vi "运维调试_CODMn.vi"() -> ()   [LabVIEW 2016, in "斯坦道CODMn新电路板.lvlib"]
uses:
  <vilib>/Utility/miscctls.llb/LVPointTypeDef.ctl
  <vilib>/Waveform/WDTFileIO.llb/Read Waveform from File.vi
  <vilib>/Utility/config.llb/NI_LVConfig.lvlib
  <vilib>/ptbypt/NI_PtbyPt.lvlib
panel:
  in  "量程下拉列表 2":enum16{"低量程", "高量程"}(ring)
  out "消解压力kPa":sgl format="%#.2f"
  out "权限等级":string
  out "总步数":i32
  out "滑动杆":u8(slide) caption="测试进度" scale=0.0..100.0
  in  "参数查询":bool
  in  "仪器校准":bool
  out "仪器版本号":string
  in  "试剂余量设置":bool
  out "试剂余量显示":sgl[][](graph)
  in  "公式切换阈值滴定数(0~9999)":dbl
  out "X0":u16
  in  "平台反控标样校准":enum16{"标液1", "标液2", "标液3"}(ring)
  in  "平台反控校准量程":enum16{"低量程1", "低量程2", "高量程1", "高量程2"}(ring)
  out "注射泵保温温度":sgl format="%#.2f"
  out "量程参数显示":T1 {"(高->低)" format="%#.6g"; "阈值(低->高)" format="%#.6g"; "下限" format="%#.6g"; "上限" format="%#.6g"}
  in  "历史波形 2":bool
  in  "返回 3":bool
  out "时间-温度":u16[](array[numeric]) caption="数组"
  out "温度波形时间":timestamp
  out "ORP滴定曲线 2":u16[](graph)
  in  "历史波形":bool
  in  "返回 2":bool
  out "滴定数-ORP值":u16[](array[numeric]) caption="数组"
  out "波形时间":timestamp
  out "ORP滴定曲线":u16[](graph)
  in  "滴定曲线":bool
  out "终点滴定数":sgl format="%#.2f"
  out "单位:":T2(ring)
  out "运行状态":T3 {"数据时间:" format="%<%y/%m/%d %H:%M:%S>T"; "仪器时间:" format="%<%y/%m/%d %H:%M:%S>T"}
  out "模块版本号":string
  in  "模型选择":cluster{"参数":u8, "测量模式":u8, "量程":u8}
  in  "校准完毕":bool
  in  "校准按钮":T4
  in  "曲线模型":T5={"标液浓度1"=0.0, "测量吸光度1"=0.0, "样品1启用"=FALSE, "标液浓度2"=0.0, "测量吸光度2"=0.0, "样品2启用"=FALSE, "标液浓度3"=0.0, "测量吸光度3"=0.0, "样品3启用"=FALSE, "标液浓度4"=0.0, "测量吸光度4"=0.0, "样品4启用"=FALSE, "标液浓度5"=0.0, "测量吸光度5"=0.0, "样品5启用"=FALSE, "模型"=enum."线性", "method"=enum."最小二乘", "精度"=7.0, "XY图"=[], "拟合公式"="", "r^2"=0.0, "零点校准时间"=timestamp(0 s since 1904-01-01), "标液校准时间1"=timestamp(0 s since 1904-01-01), "标液校准时间2"=timestamp(0 s since 1904-01-01), "标液校准时间3"=timestamp(0 s since 1904-01-01), "标液校准时间4"=timestamp(0 s since 1904-01-01)} {"标液校准时间4" format="%<%Y/%m/%d %H:%M:%S>T"; "标液校准时间3" format="%<%Y/%m/%d %H:%M:%S>T"; "标液校准时间2" format="%<%Y/%m/%d %H:%M:%S>T"; "标液校准时间1" format="%<%Y/%m/%d %H:%M:%S>T"; "零点校准时间" format="%<%Y/%m/%d %H:%M:%S>T"; "r^2" format="%.7g"; "标液浓度5" format="%#.2f"; "测量吸光度5" format="%#.0f"; "标液浓度4" format="%#.2f"; "测量吸光度4" format="%#.0f"; "标液浓度3" format="%#.2f"; "测量吸光度3" format="%#.0f"; "标液浓度2" format="%#.2f"; "测量吸光度2" format="%#.0f"; "测量吸光度1" format="%#.0f"; "标液浓度1" format="%#.2f"}
  out "公式、校准输出":T6={"公式"={"X^2"=0.0, "X"=nan, "B"=nan}, "校准"={"校准？"=FALSE, "校准点1-5"=0, "校准浓度"=0.0}}
  out "当前步骤剩余时间":sgl format="%#.2f"
  out "加热实时温度":sgl format="%#.2f"
  out "ORP值/光值":sgl format="%#.2f"
  in  "布尔":bool
  in  "流程固件":bool
  in  "公式单个写入":bool
  in  "流程路径":path=path "C:/Users/STD/Documents/斯坦道流程文件/流程.xml"
  out "字符串":string
  out "运行时间":sgl format="%#.2f"
  out "环境湿度":sgl format="%#.2g"
  out "环境温度":sgl format="%#.2g"
  out "固件版本号":string
  in  "数组":string[](array[string])
  in  "量程切换阈值写入":bool
  in  "量程切换阈值读取":bool
  in  "参数下拉列表":enum16{"CODMn"}(ring)
  in  "量程下拉列表":enum16{"低量程1", "低量程2", "高量程1", "高量程2"}(ring)
  in  "测量模式下拉列表":T7(ring)=enum."水样测量"
  in  "公式":cluster{"X^2":dbl, "X":dbl, "b":dbl}
  in  "写公式":bool
  in  "读公式":bool
  in  "返回":bool
  in  "设置":bool
  out "集成报警信息":string
  in  "定时启动":cluster{"启动":bool, "控制命令":T8, "测量参数":T9}(xcontrol)
  in  "停止":bool
  in  "手动启动":bool
  in  "单步测试":bool
  out "当前滴定数":sgl format="%#.2f"
  out "K":sgl format="%#.2f"
  out "B":sgl format="%#.2f"
  out "A":sgl format="%#.2f"
  out "多列列表框":i32(listbox)
  # "."
  # "校准时间"
  # "标液浓度"
  # "滴定数显示"
  # "标液1"
  # "标液2"
  # "标液3"
  # "零点"
  # "跨度"
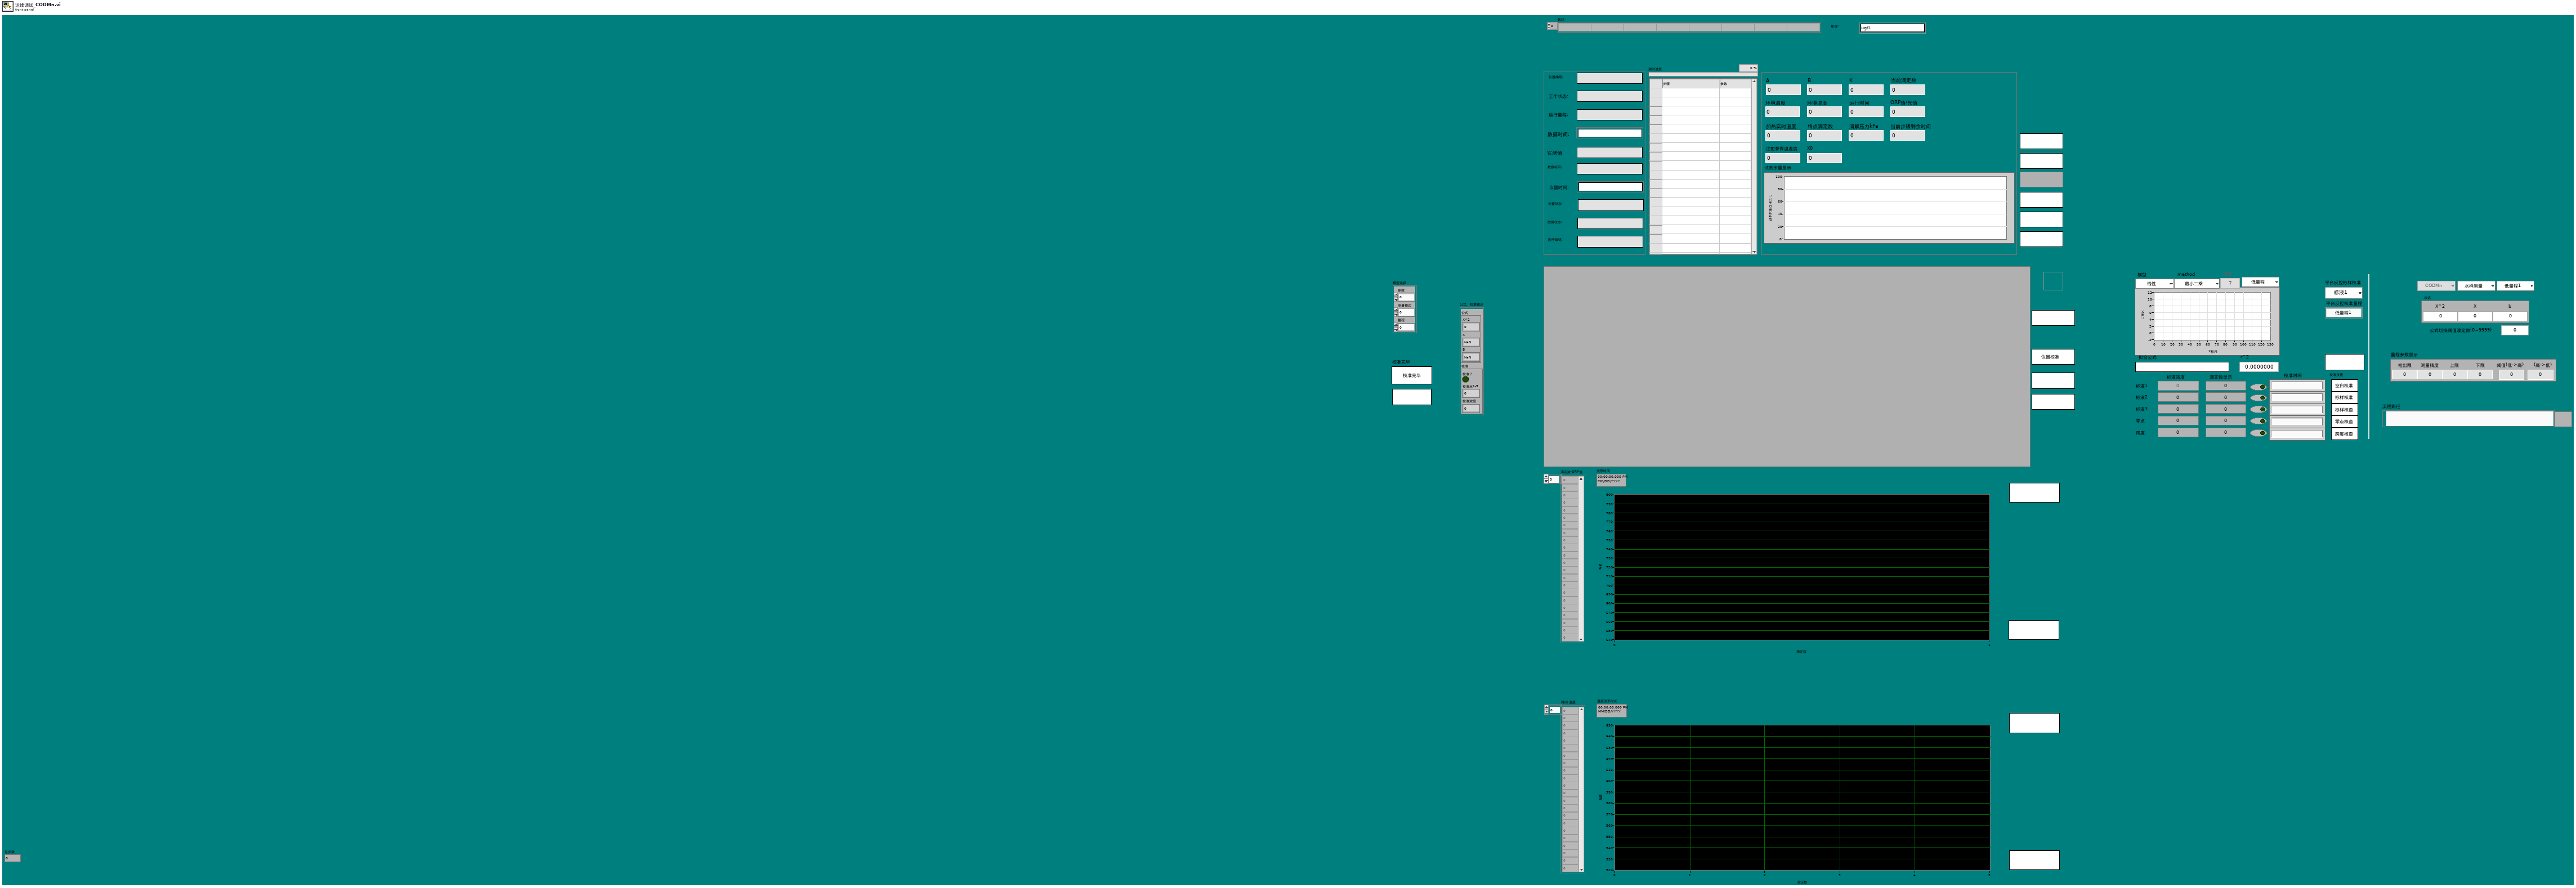
[diagram p1: front panel]
types:
  T1 = cluster{"检出限":dbl, "测量精度":dbl, "上限":dbl, "下限":dbl, "阈值(低->高)":dbl, "(高->低)":dbl}
  T2 = enum16{"ug/L", "mg/L", "ppm", "mg/m3", "cm", "ppb", "ug/m3", "%", "nmol/mol", "umol/mol", "MPN/L", "MPN/100ml", "ng/m3", "NTU", "无量纲", "ms/cm", "us/cm", "℃", "mV", "万个/L"}
  T3 = cluster{"仪器编号:":string, "工作状态:":string, "运行量程: ":string, "数据时间:":timestamp, "实测值:":string, "数据标识: ":string, "仪器时间:":timestamp, "告警状态: ":string, "故障状态:  ":string, "因子编码:":string}
  T4 = cluster{"校准1":bool, "校准2":bool, "校准3":bool, "校准4":bool, "校准5":bool}
  T5 = cluster{"标液浓度1":dbl, "测量吸光度1":dbl, "样品1启用":bool, "标液浓度2":dbl, "测量吸光度2":dbl, "样品2启用":bool, "标液浓度3":dbl, "测量吸光度3":dbl, "样品3启用":bool, "标液浓度4":dbl, "测量吸光度4":dbl, "样品4启用":bool, "标液浓度5":dbl, "测量吸光度5":dbl, "样品5启用":bool, "模型":enum32{"线性", "多项式"}, "method":enum16{"最小二乘", "最小绝对残差", "Bisquare"}, "精度":dbl, "XY图":cluster{"X Values":dbl[], "Y Values":dbl[]}[], "拟合公式":string, "r^2":dbl, "零点校准时间":timestamp, "标液校准时间1":timestamp, "标液校准时间2":timestamp, "标液校准时间3":timestamp, "标液校准时间4":timestamp}
  T6 = cluster{"公式":cluster{"X^2":dbl, "X":dbl, "B":dbl}, "校准":cluster{"校准？":bool, "校准点1-5":u16, "校准浓度":dbl}}
  T7 = enum16{"", "水样测量", "标样核查", "零点核查", "跨度核查", "空白测试", "平行样测试", "加标回收"}
  T8 = typedef "定时设置.xctl/国标控制命令.ctl" = enum16{"启动测量", "标样核查", "零点核查", "跨度核查", "空白测试", "平行样测试", "加标回收", "空白校准", "标样校准", "初始化（清洗）", "停止测试", "仪器重启", "校时", "模式设置", "测量间隔设置"}
  T9 = typedef "定时设置.xctl/测量参数.ctl" = u16
  T10 = cluster{"曲线模型":cluster{"标液浓度1":dbl, "测量吸光度1":dbl, "样品1启用":bool, "标液浓度2":dbl, "测量吸光度2":dbl, "样品2启用":bool, "标液浓度3":dbl, "测量吸光度3":dbl, "样品3启用":bool, "标液浓度4":dbl, "测量吸光度4":dbl, "样品4启用":bool, "标液浓度5":dbl, "测量吸光度5":dbl, "样品5启用":bool, "模型":enum32{"线性", "多项式"}, "method":enum16{"最小二乘", "最小绝对残差", "Bisquare"}, "精度":dbl, "XY图":cluster{"X Values":dbl[], "Y Values":dbl[]}[], "拟合公式":string, "r^2":dbl, "零点校准时间":timestamp, "标液校准时间1":timestamp, "标液校准时间2":timestamp, "标液校准时间3":timestamp, "标液校准时间4":timestamp}, "Polynomial Coefficients":dbl[]}
  T11 = cluster{"Major":u16, "Minor":u16, "Fix":u16, "Build":u16}
  T12 = typedef "NI_LVConfig.lvlib/Config Data RefNum.ctl" = refnum<k1>
  T13 = cluster{"测量量程":sgl, "测量检出限":sgl, "测量精度":sgl, "测量间隔":sgl, "消解温度":sgl, "消解时长":sgl, "三项式系数":sgl, "二次多项式系数":sgl, "曲线斜率":sgl, "曲线截距":sgl, "线性相关系数":sgl, "空白校准时间":timestamp, "标样校准时间":timestamp, "测量信号值":sgl, "稀释倍数":sgl, "量程系数":sgl}
  T14 = typedef "LVPointTypeDef.ctl" = cluster{"Horizontal":i16, "Vertical":i16}
  T15 = enum32{"Bad", "Idle", "Run top level", "Running"}
  T16 = cluster{"Polynomial Coefficients[0]":dbl, "Polynomial Coefficients[1]":dbl, "Polynomial Coefficients[2]":dbl}
  T17 = cluster{"检出限":dbl, "测量精度":dbl, "上限":dbl, "下限":dbl, "阈值（低->高）":dbl, "阈值（高->低）":dbl}
  T18 = cluster{"系统时间":timestamp, "工作状态":u16, "测量模式":enum16{"待机", "连续模式", "周期模式", "定点模式", "受控模式", "手动模式"}, "告警代码":u16, "故障代码":u16, "日志代码":u16, "软件版本":u16, "A":sgl, "B":sgl, "K":sgl, "当前滴定数":sgl, "T":sgl, "H":sgl, "id":u16, "flowid":u16, "量程":u16, "加热实时温度":sgl, "当前ORP值":sgl, "运行时间":sgl, "当前步骤剩余时间":sgl, "结束滴定数":sgl, "注射泵保温温度":sgl, "匹配滴定数X0":u16, "X^2":sgl, "X":sgl, "B 2":sgl, "光值1":sgl, "光值2":sgl, "光值3":sgl, "光值4":sgl, "光值5":sgl, "光值6":sgl, "光值7":sgl, "光值8":sgl}
  T19 = cluster{"因子编码":u32, "单位":u16, "标样参考值":sgl, "水样数据时间":timestamp, "水样实测值":sgl, "水样数据标识":string, "标样数据时间":timestamp, "标样实测值":sgl, "标样数据标识":string, "空白数据时间":timestamp, "空白实测值":sgl, "空白数据标识":string, "零点核查数据时间":timestamp, "零点核查实测值":sgl, "零点核查数据标识":string, "跨度核查数据时间":timestamp, "跨度核查实测值":sgl, "跨度核查数据标识":string, "加标回收数据时间":timestamp, "加标回收实测值":sgl, "加标回收数据标识":string, "平行样数据时间":timestamp, "平行样实测值":sgl, "平行样数据标识":string, "F0":sgl, "F1":sgl, "F2":sgl, "F3":sgl, "F4":sgl, "F5":sgl, "F6":sgl, "F7":sgl, "温度":sgl, "湿度":sgl, "X值":sgl, "fidrange":u16}
  T20 = cluster{"时间标识":timestamp, "设备":string, "日志信息":string, "流程参数":string}
  T21 = cluster{"时间标识":timestamp, "设备":string, "日志信息":string, "备注":string}
  T22 = typedef "LVRowAndColumnUnsignedTypeDef.ctl" = cluster{"Row":u32, "Column":u32}
  T23 = enum8{"Enabled", "Disabled", "Disabled and Grayed Out"}
  T24 = enum16{"空闲", "水样测试", "标样核查", "零点核查", "跨度核查", "空白测试", "平行样测试", "加标回收", "空白校准", "标样校准", "初始化（清洗）"}
  T25 = cluster{"站号":u16, "量程切换":enum32{"H", "L", "AUTO"}, "控制命令":u16, "模式设置":enum16{"待机", "连续模式", "周期模式", "定点模式", "受控模式", "手动模式"}, "测量间隔":u16}
  T26 = cluster{"参数下拉列表":enum16{"CODMn"}, "测量模式下拉列表":enum16{"", "水样测量", "标样核查", "零点核查", "跨度核查", "空白测试", "平行样测试", "加标回收"}, "量程下拉列表":enum16{"低量程1", "低量程2", "高量程1", "高量程2"}}
  T27 = cluster{"测量量程":dbl, "测量精度":dbl, "测量间隔":dbl, "消解温度":dbl, "消解时长":dbl, "空白校准时间":timestamp, "曲线截距":dbl, "曲线斜率":dbl, "测量检出限":dbl, "测量信号值":dbl, "线性相关系数":dbl, "二次多项式系数":dbl, "标样校准时间":timestamp, "稀释倍数":dbl, "三项式系数":dbl, "空白标定系数":dbl, "量程系数":dbl, "F0/ORPA":dbl, "F1/ORPB":dbl, "F2/ORPK":dbl, "F3":dbl, "F4":dbl, "F5":dbl, "F6":dbl, "F7":dbl, "X0/滴定数":dbl, "量程":dbl}
  T28 = cluster{"跨度值":dbl, "零点标准液浓度":dbl, "跨度标准液浓度":dbl, "标准液标准浓度":dbl, "零点标准液偏差":dbl, "跨度标准液偏差":dbl, "标准液标准偏差":dbl}
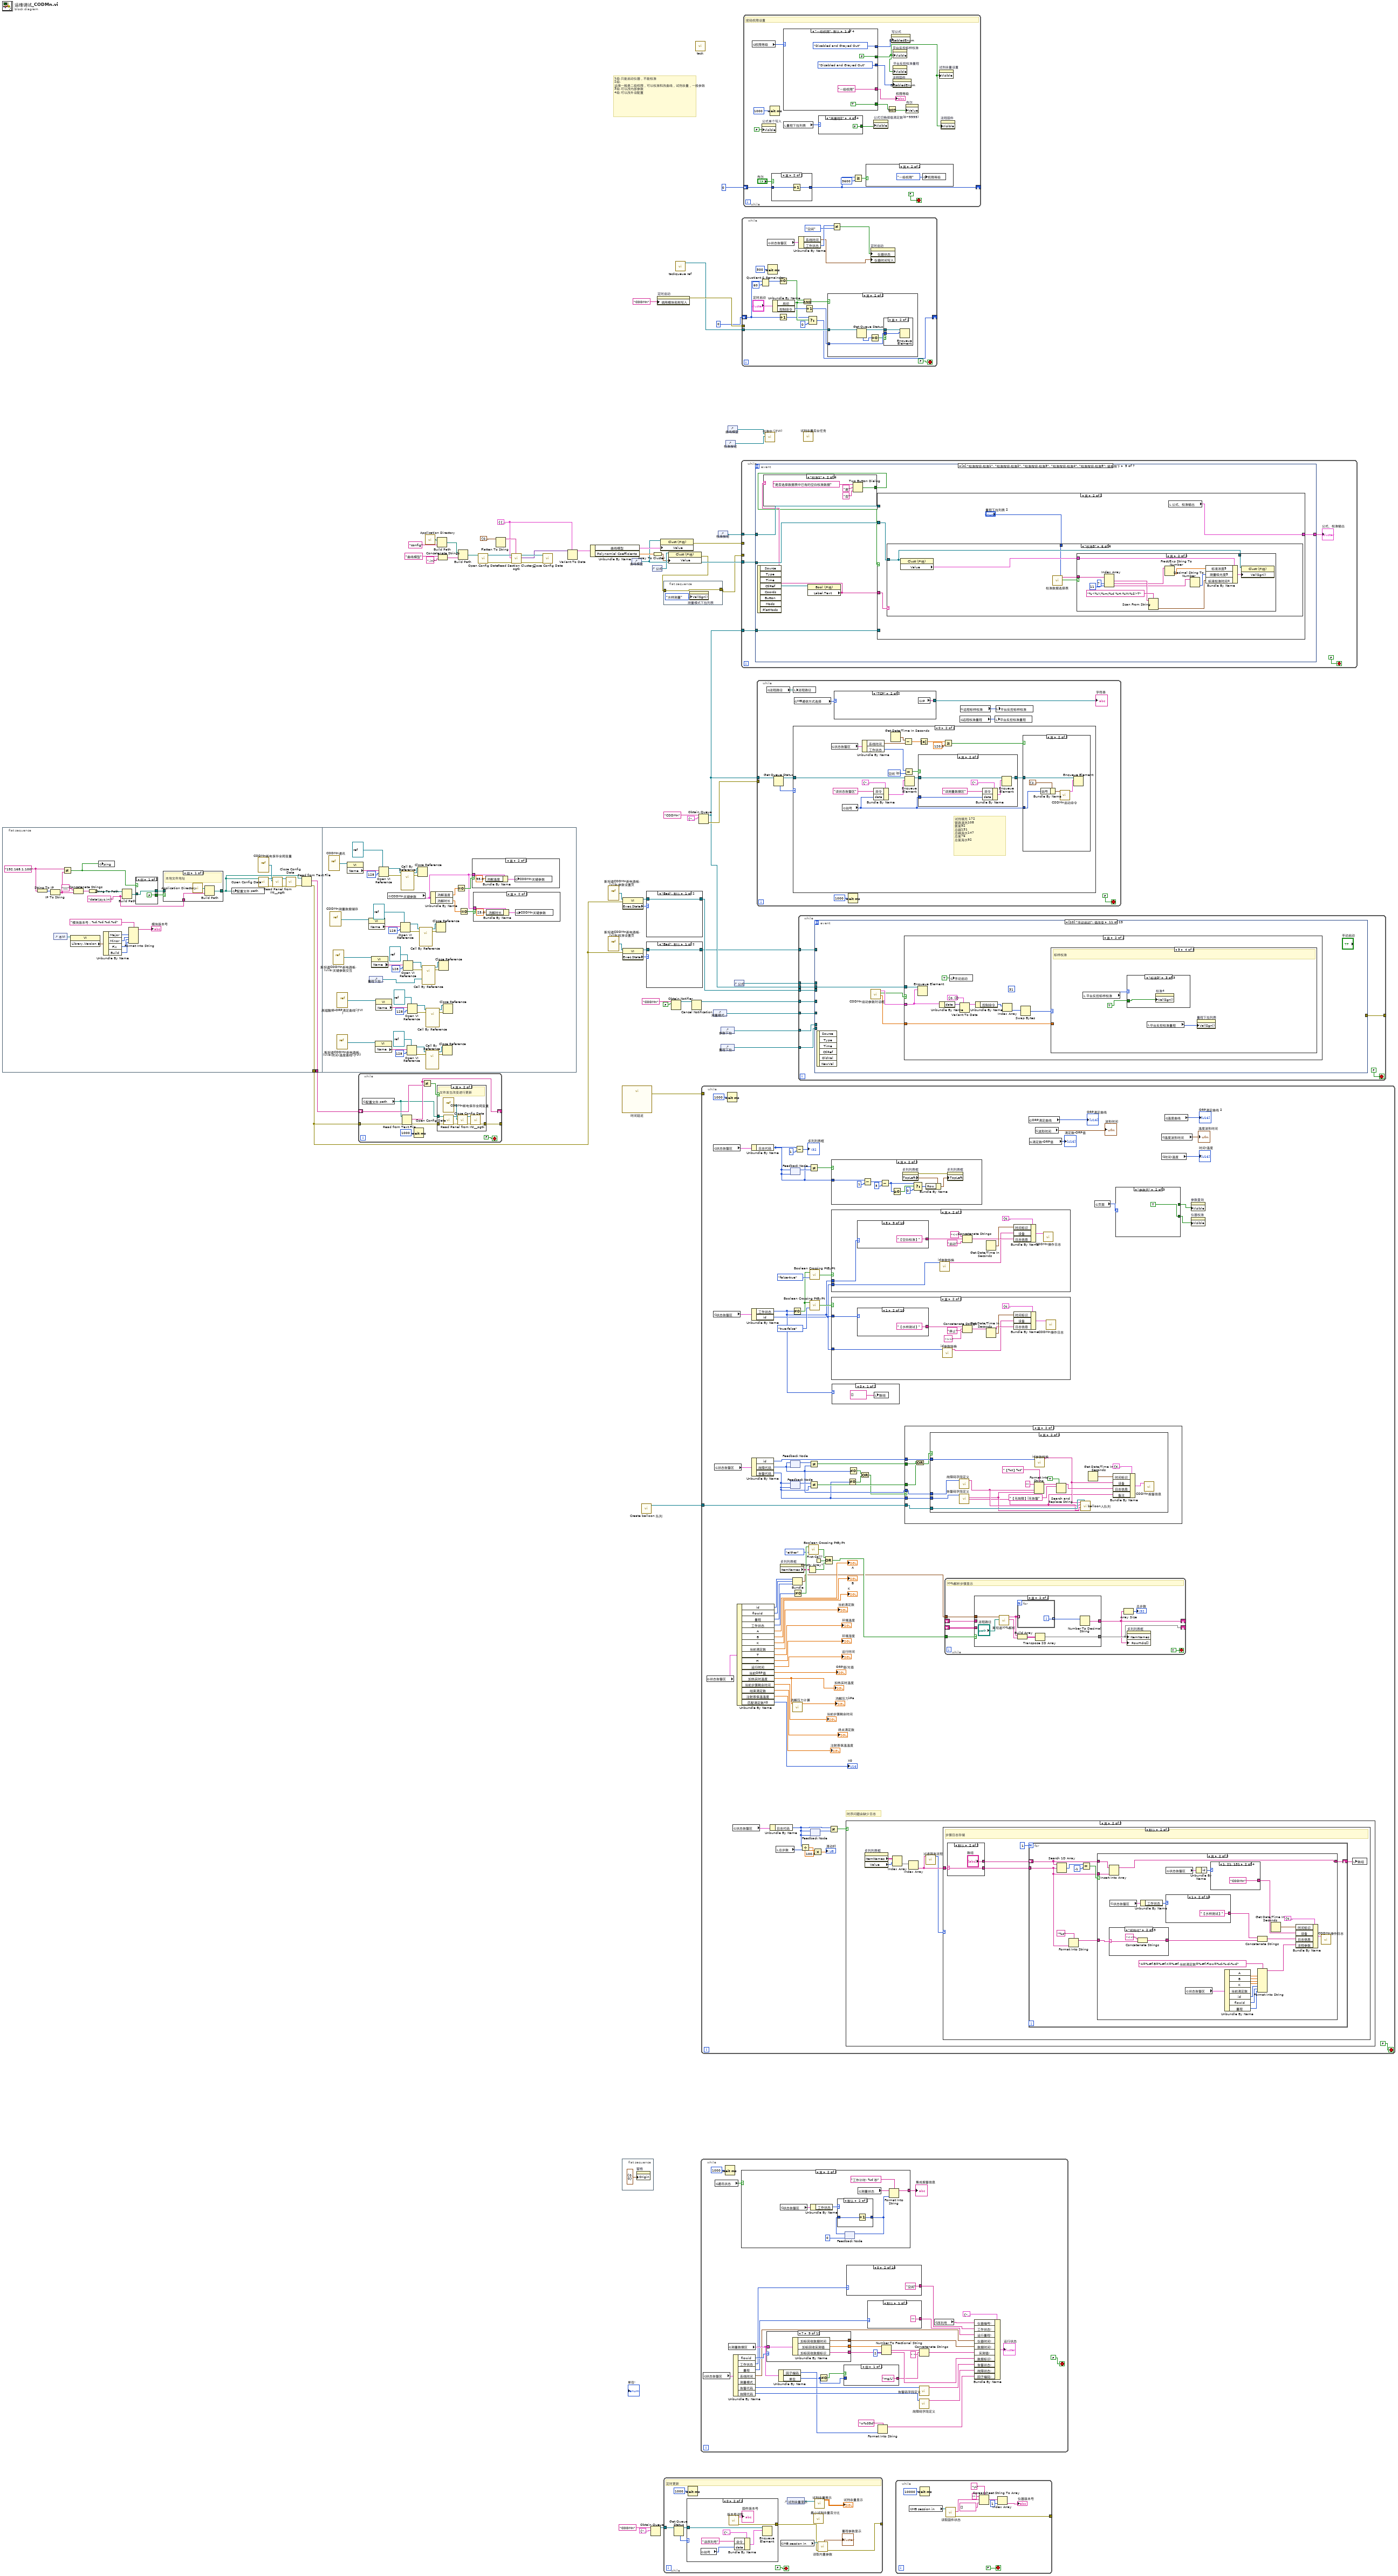
[diagram p0: block diagram]
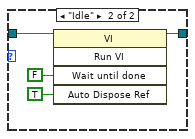
[diagram p2: hidden frame]
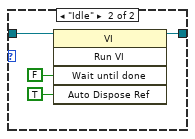
[diagram p3: hidden frame]
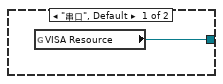
[diagram p8: hidden frame]
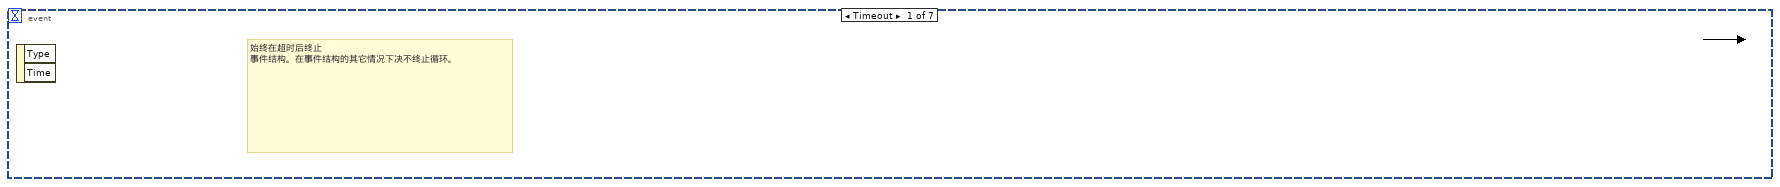
[diagram p12: hidden frame]
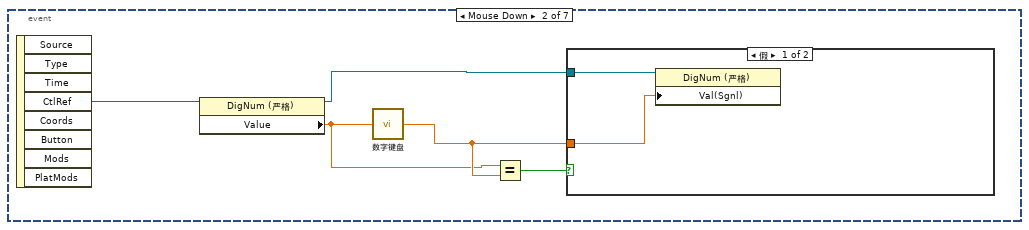
[diagram p13: hidden frame]
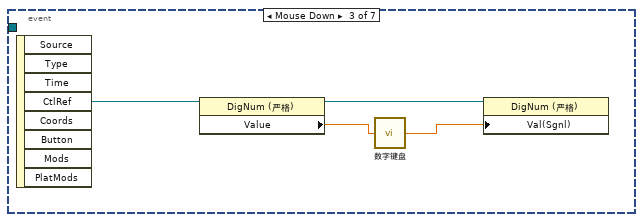
[diagram p15: hidden frame]
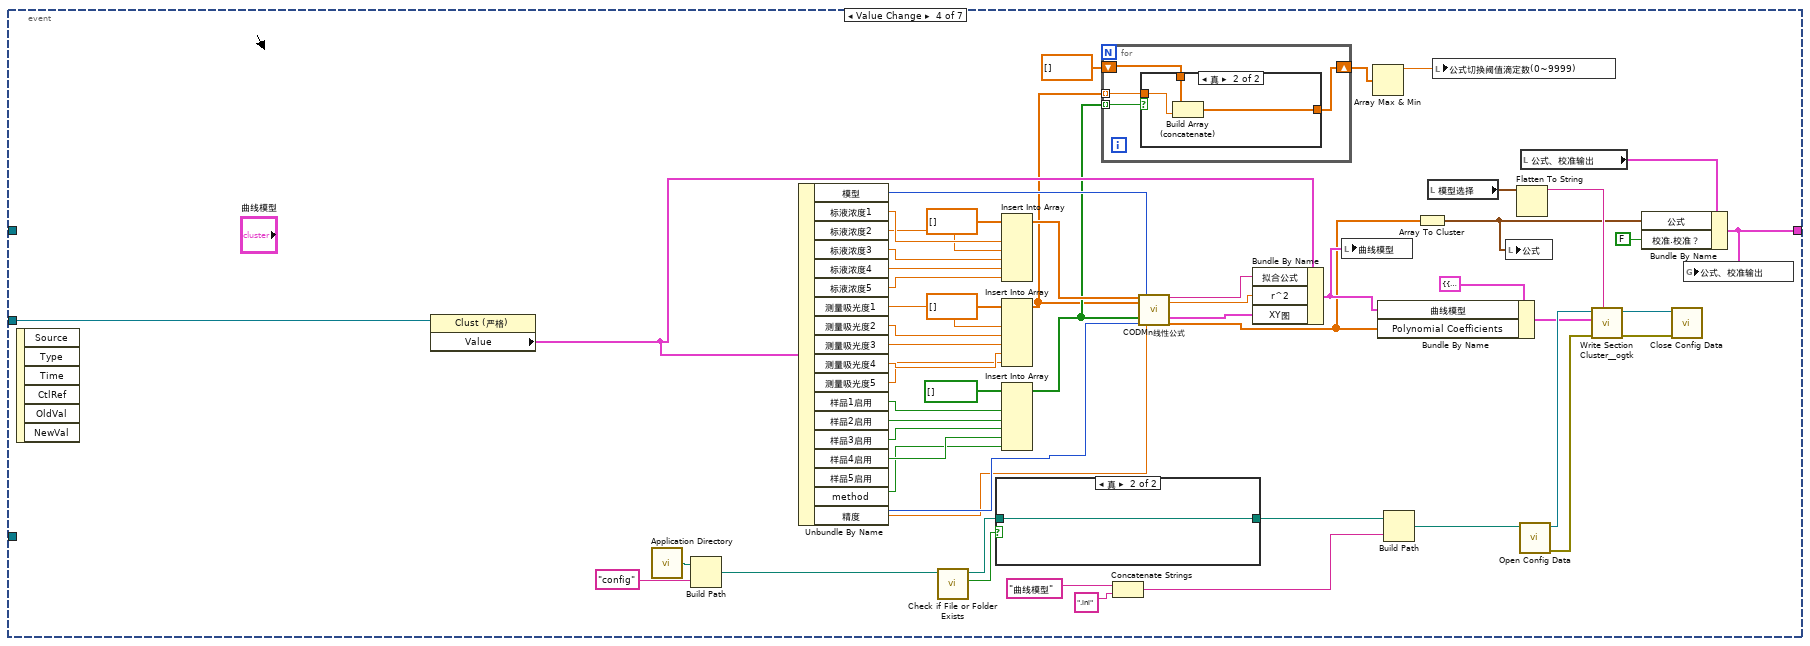
[diagram p16: hidden frame]
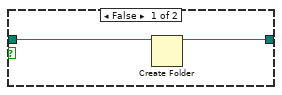
[diagram p18: hidden frame]
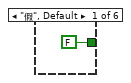
[diagram p19: hidden frame]
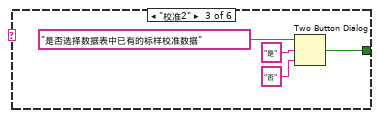
[diagram p20: hidden frame]
diagram:
  w26 = T10 {"曲线模型"={"标液浓度1"=0.0, "测量吸光度1"=0.0, "样品1启用"=FALSE, "标液浓度2"=0.0, "测量吸光度2"=0.0, "样品2启用"=FALSE, "标液浓度3"=0.0, "测量吸光度3"=0.0, "样品3启用"=FALSE, "标液浓度4"=0.0, "测量吸光度4"=0.0, "样品4启用"=FALSE, "标液浓度5"=0.0, "测量吸光度5"=0.0, "样品5启用"=FALSE, "模型"=enum."线性", "method"=enum."最小二乘", "精度"=7.0, "XY图"=[], "拟合公式"="", "r^2"=0.0, "零点校准时间"=timestamp(0 s since 1904-01-01), "标液校准时间1"=timestamp(0 s since 1904-01-01), "标液校准时间2"=timestamp(0 s since 1904-01-01), "标液校准时间3"=timestamp(0 s since 1904-01-01), "标液校准时间4"=timestamp(0 s since 1904-01-01)}, "Polynomial Coefficients"=[]} ("输出簇")
  # "1级.只能启动仪器，不能校准\n2级.运维一般是二级权限，可以校准和改曲线，试剂余量，一般参数\n3级.可以改内部参数\n4级.可以改外设配置"
  n1 = flat-sequence {
    tunnel: [w61] -> w3
    tunnel: [w60] -> w43
    frame #0 {
      w81 = "data\\sys.ini" ("名称或相对路径")
      w73 = "192.168.1.100" ("名称")
      n2 = String To IP(1:w73) -> (0:w80:u32)
      n3 = IP To String(2:w80) -> (0:w77:string)  [unwired: 1 in]
      n4 = control-ref of="本VI"() -> (w71:refnum<vi>)
      n5 = Not Equal?(x=w73, y=w77) -> (x != y?=w82:bool)
      n6 = property class="VI"(reference=w71) -> ("Library.Version"=w70:T11)  [unwired: 1 in, 2 out]
      n7 = Concatenate Strings("\\\\" ("字符串"), w77) -> (w78:string)
      n8 = String To Path(string=w78) -> (path=w72:path)
      n9 = global write "VARCODMn全局变量.vi" "ping"(w82) -> ()
      n10 = Unbundle By Name(w70) -> ("Major"=w68:u16, "Minor"=w67:u16, "Fix"=w66:u16, "Build"=w65:u16)
      n11 = Build Path(base path=w72, name or relative path=w81) -> (appended path=w76:path)
      n12 = Format Into String(format string="模块版本号：%d.%d.%d.%d" ("格式字符串"), w68, w67, w66, w65) -> (resulting string=→"模块版本号":string)  [unwired: 2 in, 1 out]
      n13 = case shown="假" w82 {
        tunnel: w76 -> [w88 w92]
        tunnel: [w88 w91] -> w75
        tunnel: [FALSE w90] -> w74
        frame False {
        }
        frame True {
          n14 = call <vilib>:"Check if File or Folder Exists.vi"("path"=w92) -> ("file or folder exists?"=w90:bool, "dup path"=w91:path)  [unwired: 8 in, 1 out]
        }
      }
      n15 = case shown="假" w74 {
        tunnel: w75 -> [_ w96]
        tunnel: [w94 w96] -> w63
        tunnel: w81 -> [w93 _]
        frame False {
          # "本地文件地址"
          n16 = call <vilib>:"Application Directory.vi"() -> ("Application Directory"=w95:path)
          n17 = Build Path(base path=w95, name or relative path=w93) -> (appended path=w94:path)
        }
        frame True {
          # "网络共享地址"
        }
      }
      n18 = global write "VARCODMn全局变量.vi" "配置文件 path"(w63) -> ()
      n19 = vi-ref "CODMn断电保存全局变量.vi"() -> (w86:refnum<vi>)
      n20 = call <vilib>:"Open Config Data.vi"("configuration file path"=w63) -> ("error out"=w84:errorcluster, "refnum"=w87:T12)  [unwired: 8 in, 1 out]
      n21 = call <userlib>:"Read Panel from INI__ogtk.vi"("error in (no error)"=w84, "VI ref"=w86, "refnum"=w87) -> ("error out"=w83:errorcluster, "refnum out"=w85:T12)  [unwired: 7 in]
      n22 = call <vilib>:"Close Config Data.vi"("error in (no error)"=w83, "refnum"=w85) -> ("error out"=w62:errorcluster)  [unwired: 8 in, 1 out]
      n23 = Read from Text File(file (use dialog)=w63, error in=w62) -> (text=w60:string, error out=w61:errorcluster)  [unwired: 2 in, 2 out]
    }
    frame #1 {
      n24 = vi-ref "CODMn通讯.vi"() -> (w110:refnum<vi>)
      n25 = vi-ref "CODMn测量数据储存.vi"() -> (w142:refnum<vi>)
      n26 = vi-ref "斯坦道CODMn新电路板.lvlib:关键参数交互.vi"() -> (w128:refnum<vi>)
      n27 = vi-ref "斯坦道CODMn新电路板.lvlib:时间-温度曲线(子VI).vi"() -> (w112:refnum<vi>)
      n28 = vi-ref "高锰酸钾-ORP滴定曲线(子VI).vi"() -> (w125:refnum<vi>)
      n29 = property class="VI"(reference=w110) -> ("Name"=w109:string)  [unwired: 1 in, 2 out]
      n30 = property class="VI"(reference=w142) -> ("Name"=w135:string)  [unwired: 1 in, 2 out]
      n31 = control-ref of="量程下拉列表"() -> (w102:refnum<vi>)
      n32 = property class="VI"(reference=w128) -> ("Name"=w134:string)  [unwired: 1 in, 2 out]
      n33 = property class="VI"(reference=w112) -> ("Name"=w118:string)  [unwired: 1 in, 2 out]
      n34 = property class="VI"(reference=w125) -> ("Name"=w119:string)  [unwired: 1 in, 2 out]
      n35 = Open VI Reference(type specifier VI Refnum (for type only)=refnum<vi> refnum, vi path=w109, options=128 ("选项")) -> (vi reference=w107:refnum<vi>, error out=w105:errorcluster)  [unwired: 3 in]
      n36 = global read "CODMn断电保存全局变量.vi" "CODMn关键参数"() -> (w97:T13)
      n37 = Open VI Reference(type specifier VI Refnum (for type only)=refnum<vi> refnum, vi path=w135, options=128 ("选项")) -> (vi reference=w137:refnum<vi>, error out=w139:errorcluster)  [unwired: 3 in]
      n38 = call-by-ref "?"(reference=w107, error in=w105) -> (reference out=w103:refnum<vi>, error out=w104:errorcluster)  [unwired: 12 in]
      n39 = Open VI Reference(type specifier VI Refnum (for type only)=refnum<vi> refnum, vi path=w134, options=128 ("选项")) -> (vi reference=w132:refnum<vi>, error out=w131:errorcluster)  [unwired: 3 in]
      n40 = Open VI Reference(type specifier VI Refnum (for type only)=refnum<vi> refnum, vi path=w118, options=128 ("选项")) -> (vi reference=w116:refnum<vi>, error out=w115:errorcluster)  [unwired: 3 in]
      n41 = Open VI Reference(type specifier VI Refnum (for type only)=refnum<vi> refnum, vi path=w119, options=128 ("选项")) -> (vi reference=w121:refnum<vi>, error out=w122:errorcluster)  [unwired: 3 in]
      n42 = Close Reference(reference=w103, error in (no error)=w104) -> ()  [unwired: 1 out]
      n43 = call-by-ref "?"(reference=w137, error in=w139) -> (reference out=w141:refnum<vi>, error out=w140:errorcluster)  [unwired: 12 in]
      n44 = call-by-ref "?"(reference=w132, error in=w131, "量程下拉列表"=w102) -> (reference out=w129:refnum<vi>, error out=w130:errorcluster)  [unwired: 11 in]
      n45 = call-by-ref "?"(reference=w116, error in=w115) -> (reference out=w113:refnum<vi>, error out=w114:errorcluster)  [unwired: 12 in]
      n46 = call-by-ref "?"(reference=w121, error in=w122) -> (reference out=w124:refnum<vi>, error out=w123:errorcluster)  [unwired: 12 in]
      n47 = Unbundle By Name(w97) -> ("消解温度"=w101:sgl, "消解时长"=w98:sgl)
      n48 = Close Reference(reference=w141, error in (no error)=w140) -> ()  [unwired: 1 out]
      n49 = Close Reference(reference=w129, error in (no error)=w130) -> ()  [unwired: 1 out]
      n50 = Close Reference(reference=w113, error in (no error)=w114) -> ()  [unwired: 1 out]
      n51 = Close Reference(reference=w124, error in (no error)=w123) -> ()  [unwired: 1 out]
      n52 = Equal To 0?(x=w101) -> (x = 0?=w100:bool)
      n53 = Equal To 0?(x=w98) -> (x = 0?=w99:bool)
      n54 = case shown="真" w100 {
        tunnel: w97 -> [_ w148]
        frame False {
        }
        frame True {
          n55 = Bundle By Name(cluster=w148, "消解温度"=sgl 95.0) -> (w147:T13)
          n56 = global write "CODMn断电保存全局变量.vi" "CODMn关键参数"(w147) -> ()
        }
      }
      n57 = case shown="真" w99 {
        tunnel: w97 -> [_ w145]
        frame False {
        }
        frame True {
          n58 = Bundle By Name(cluster=w145, "消解时长"=sgl 25.0) -> (w144:T13)
          n59 = global write "CODMn断电保存全局变量.vi" "CODMn关键参数"(w144) -> ()
        }
      }
    }
  }
  n60 = while {
    tunnel: [w156] -> _
    shift-right: [w151] -> _
    shift-left: w43 -> [w154]
    tunnel: w3 -> [w152]
    stop <- FALSE stop-if-true
    n61 = global read "VARCODMn全局变量.vi" "配置文件 path"() -> (w149:path)
    n62 = Read from Text File(file (use dialog)=w149, error in=w152) -> (text=w151:string, error out=w150:errorcluster)  [unwired: 2 in, 2 out]
    n63 = Wait (ms)(milliseconds to wait=u32 1000 ("等待时间（毫秒）")) -> ()  [unwired: 1 out]
    n64 = Not Equal?(x=w151, y=w154) -> (x != y?=w153:bool)
    n65 = case shown="真" w153 {
      tunnel: [w158 w162] -> w156
      tunnel: w149 -> [_ w161]
      tunnel: w150 -> [w158 w160]
      frame False {
      }
      frame True {
        # "文件发生改变进行更新"
        n66 = vi-ref "CODMn断电保存全局变量.vi"() -> (w159:refnum<vi>)
        n67 = call <vilib>:"Open Config Data.vi"("error in (no error)"=w160, "configuration file path"=w161) -> ("error out"=w166:errorcluster, "refnum"=w165:T12)  [unwired: 7 in, 1 out]
        n68 = call <userlib>:"Read Panel from INI__ogtk.vi"("error in (no error)"=w166, "VI ref"=w159, "refnum"=w165) -> ("error out"=w164:errorcluster, "refnum out"=w163:T12)  [unwired: 7 in]
        n69 = call <vilib>:"Close Config Data.vi"("error in (no error)"=w164, "refnum"=w163) -> ("error out"=w162:errorcluster)  [unwired: 8 in, 1 out]
      }
    }
  }
  n70 = call <vilib>:"Application Directory.vi"() -> ("Application Directory"=w36:path)
  n71 = Build Path(base path=w36, name or relative path="config" ("名称或相对路径")) -> (appended path=w34:path)
  n72 = Concatenate Strings("曲线模型" ("字符串"), ".ini" ("字符串")) -> (w32:string)
  n73 = Build Path(base path=w34, name or relative path=w32) -> (appended path=w37:path)
  n74 = call <vilib>:"Open Config Data.vi"("configuration file path"=w37) -> ("error out"=w40:errorcluster, "refnum"=w41:T12)  [unwired: 8 in, 1 out]
  n75 = Flatten To String(anything=cluster{"参数":u8, "测量模式":u8, "量程":u8} {"参数"=0, "测量模式"=0, "量程"=0} ("模型选择")) -> (data string=w30:string)  [unwired: 3 in, 2 out]
  n76 = call <userlib>:"Read Section Cluster__ogtk.vi"("section (optional)"=w30, "error in (no error)"=w40, "Section Formatted Cluster Type"=w26, "refnum"=w41) -> ("error out"=w38:errorcluster, "Section Formatted Cluster"=w31:variant, "dup refnum"=w39:T12)  [unwired: 3 in, 2 out]
  n77 = call <vilib>:"Close Config Data.vi"("error in (no error)"=w38, "refnum"=w39) -> ()  [unwired: 8 in, 2 out]
  n78 = Variant To Data(type=w26, Variant=w31) -> (data=w28:T10)  [unwired: 1 in, 1 out]
  n79 = Unbundle By Name(w28) -> ("曲线模型"=w27:T5, "Polynomial Coefficients"=w25:dbl[])
  n80 = vi-ref "斯坦道CODMn新电路板.lvlib:参数设置页.vi"() -> (w8:refnum<vi>)
  n81 = vi-ref "斯坦道CODMn新电路板.lvlib:校准设置页.vi"() -> (w11:refnum<vi>)
  n82 = call "时间延迟"() -> ("error out"=w52:errorcluster)  [unwired: 11 in]
  n83 = flat-sequence {
    frame #0 {
      n84 = property on="窗格" class="Pane"("Origin"=T14 {"Horizontal"=0, "Vertical"=0} ("原点")) -> ()  [unwired: 2 in, 2 out]
    }
  }
  n85 = property class="VI"(reference=w8, error in=w3) -> (reference out=w6:refnum<vi>, "Exec.State"=w7:T15)  [unwired: 1 out]
  n86 = property class="VI"(reference=w11, error in=w3) -> (reference out=w9:refnum<vi>, "Exec.State"=w10:T15)  [unwired: 1 out]
  n87 = control-ref of="曲线模型"() -> (w23:refnum<vi>)
  n88 = call "Create balloon 队列.vi"() -> ("队列输出"=w42:refnum<queue>)  [unwired: 11 in]
  n89 = case shown="\"Bad\", 默认" w7 {
    tunnel: w6 -> [w168 w172]
    tunnel: [w168 w169] -> w5
    frame "Bad", Default {
    }
    frame "Idle" {
      n90 = invoke class="VI" method="Run VI"(reference=w172, "Wait until done"=FALSE ("结束前等待"), "Auto Dispose Ref"=TRUE ("自动销毁引用")) -> (reference out=w169:refnum<vi>)  [unwired: 2 in, 4 out]
    }
  }
  n91 = case shown="\"Bad\", 默认" w10 {
    tunnel: w9 -> [w173 w177]
    tunnel: [w173 w174] -> w4
    frame "Bad", Default {
    }
    frame "Idle" {
      n92 = invoke class="VI" method="Run VI"(reference=w177, "Wait until done"=FALSE ("结束前等待"), "Auto Dispose Ref"=TRUE ("自动销毁引用")) -> (reference out=w174:refnum<vi>)  [unwired: 2 in, 4 out]
    }
  }
  n93 = Obtain Queue(name (unnamed)="CODMn" ("名称（未命名）"), element data type=cluster{"命令":string, "data":variant} {"命令"="", "data"=variant}) -> (queue out=w16:refnum<queue>)  [unwired: 3 in, 2 out]
  n94 = control-ref of="公式"() -> (w22:refnum<vi>)
  n95 = Array To Cluster(array=w25) -> (cluster=w21:T16)
  n96 = property on="定时启动" class="定时设置 (严格)"("调用模块名称写入"="CODMn" ("引用参数")) -> (error out=w15:errorcluster)  [unwired: 2 in, 1 out]
  n97 = property class="Clust (严格)"(reference=w23, "Value"=w27) -> (error out=w20:errorcluster)  [unwired: 1 in, 1 out]
  n98 = flat-sequence {
    tunnel: w13 -> [w178]
    tunnel: [w178] -> w12
    frame #0 {
      n99 = property on="测量模式下拉列表" class="Enum (严格)"("Val(Sgnl)"=T7."水样测量" ("值(信号)")) -> ()  [unwired: 2 in, 2 out]
    }
  }
  n100 = while {
    tunnel: w16 -> [w189]
    tunnel: [w182] -> _
    stop <- FALSE stop-if-true
    # "定时更新"
    n101 = Get Queue Status(queue=w189) -> (queue out=w187:refnum<queue>, # elements in queue=w186:i32)  [unwired: 2 in, 6 out]
    n102 = case shown="0" w186 {
      tunnel: [_ w194] -> w183
      tunnel: w187 -> [_ w193]
      frame Default {
      }
      frame 0 {
        n103 = global read "CODMn断电保存全局变量.vi" "站号"() -> (w192:u16)
        n104 = call "版本号读取.vi"() -> ("error out"=w194:errorcluster, "固件版本号"=→"固件版本号":string)  [unwired: 10 in]
        n105 = Bundle By Name(cluster=cluster{"命令":string, "data":variant} {"命令"="", "data"=variant} ("元素"), "命令"="读序列号", "data"=w192) -> (w195:cluster{"命令":string, "data":variant})
        n106 = Enqueue Element(queue=w193, element=w195) -> ()  [unwired: 2 in, 3 out]
      }
    }
    n107 = Wait (ms)(milliseconds to wait=u32 1000 ("等待时间（毫秒）")) -> ()  [unwired: 1 out]
    n108 = global read "VARCODMn全局变量.vi" "MB session in"() -> (w185:refnum<class "MB_Master.lvclass">)
    n109 = control-ref of="试剂余量显示"() -> (w180:refnum<vi>)
    n110 = call "最小试剂余量百分比.vi"() -> ()  [unwired: 12 in]
    n111 = call "试剂余量展示.vi"("波形图 2"=w180) -> ("波形图"=→"试剂余量显示":sgl[][])  [unwired: 10 in]
    n112 = call "读取内置参数.vi"("error in (no error)"=w183, "MB session in"=w185) -> ("error out"=w182:errorcluster, "量程参数读取"=→"量程参数显示":T17)  [unwired: 5 in, 3 out]
  }
  n113 = property class="Clust (严格)"(reference=w22, "Value"=w21) -> (error out=w13:errorcluster)  [unwired: 1 in, 1 out]
  n114 = Obtain Notifier(name (unnamed)="CODMn" ("名称（未命名）"), notification data type=FALSE) -> (notifier out=w49:refnum<notifier>)  [unwired: 2 in, 2 out]
  n115 = call "taskqueue ref.vi"() -> ("队列输出"=w2:refnum<queue>)  [unwired: 10 in, 1 out]
  n116 = Cancel Notification(0:w49) -> (8:w48:refnum<notifier>)  [unwired: 1 in, 2 out]
  n117 = call "task.vi"() -> ()  [unwired: 12 in]
  n118 = Obtain Queue(name (unnamed)="CODMn" ("名称（未命名）"), element data type=cluster{"命令":string, "data":variant} {"命令"="", "data"=variant}) -> (queue out=w46:refnum<queue>, error out=w57:errorcluster)  [unwired: 3 in, 1 out]
  n119 = while {
    stop <- FALSE stop-if-true
    n120 = global read "VARCODMn全局变量.vi" "状态告警区"() -> (w225:T18)
    n121 = global read "VARCODMn全局变量.vi" "通讯状态"() -> (w227:bool)
    n122 = Wait (ms)(milliseconds to wait=u32 1000 ("等待时间（毫秒）")) -> ()  [unwired: 1 out]
    n123 = global read "VARCODMn全局变量.vi" "测量数据区"() -> (w223:T19)
    n124 = Unbundle By Name(w225) -> ("flowid"=w224:u16, "工作状态"=w221:u16, "量程"=w219:u16, "系统时间"=w217:timestamp, "告警代码"=w207:u16, "故障代码"=w205:u16)  [unwired: 1 out]
    n125 = case shown="真" w227 {
      tunnel: ["通讯异常" ("集成报警信息") w305] -> w226
      frame False {
      }
      frame True {
        n126 = global read "VARCODMn全局变量.vi" "状态告警区"() -> (w311:T18)
        n127 = Unbundle By Name(w311) -> ("工作状态"=w310:u16)
        n128 = feedback #1(0) -> (w308:i32)
        n129 = case shown="默认" w310 {
          tunnel: w308 -> [_ w313]
          tunnel: [_ w312] -> w306
          frame 0 {
          }
          frame Default {
            n130 = Increment(x=w313) -> (x+1=w312:i32)
          }
        }
        n131 = feedback-in #1(w306) -> ()
        n132 = global read "VARCODMn全局变量.vi" "测量状态"() -> (w304:string)
        n133 = Format Into String(format string="工作计时: %d 秒" ("格式字符串"), initial string=w304, w306) -> (resulting string=w305:string)  [unwired: 1 in, 1 out]
      }
    }
    "集成报警信息" <- w226
    n134 = case shown="7" w224 {
      selector: w224 -> [w256 _ _ _ _ _ _ _ _ _ _ _]
      tunnel: [_ w262 w266 w270 w274 w278 w282 w286 w290 w293 w297 w302] -> w214
      tunnel: [_ w260 w265 w269 w273 w277 w281 w284 w289 w292 w296 w301] -> w209
      tunnel: [_ w259 w264 w268 w272 w276 w280 w283 w288 w291 w295 w300] -> w208
      tunnel: w223 -> [_ w261 w263 w267 w271 w275 w279 w285 w287 w294 w298 w299]
      frame Default {
        n135 = Format Into String(format string="%d" ("格式字符串"), initial string="未知" ("工作状态"), w256) -> ()  [unwired: 1 in, 2 out]
      }
      frame 0 {
        n136 = Unbundle By Name(w261) -> ("水样数据时间"=w262:timestamp, "水样实测值"=w260:sgl, "水样数据标识"=w259:string)
      }
      frame 1 {
        n137 = Unbundle By Name(w263) -> ("水样数据时间"=w266:timestamp, "水样实测值"=w265:sgl, "水样数据标识"=w264:string)
      }
      frame 2 {
        n138 = Unbundle By Name(w267) -> ("标样数据时间"=w270:timestamp, "标样实测值"=w269:sgl, "标样数据标识"=w268:string)
      }
      frame 3 {
        n139 = Unbundle By Name(w271) -> ("零点核查数据时间"=w274:timestamp, "零点核查实测值"=w273:sgl, "零点核查数据标识"=w272:string)
      }
      frame 4 {
        n140 = Unbundle By Name(w275) -> ("跨度核查数据时间"=w278:timestamp, "跨度核查实测值"=w277:sgl, "跨度核查数据标识"=w276:string)
      }
      frame 5 {
        n141 = Unbundle By Name(w279) -> ("空白数据时间"=w282:timestamp, "空白实测值"=w281:sgl, "空白数据标识"=w280:string)
      }
      frame 6 {
        n142 = Unbundle By Name(w285) -> ("平行样数据时间"=w286:timestamp, "平行样实测值"=w284:sgl, "平行样数据标识"=w283:string)
      }
      frame 7 {
        n143 = Unbundle By Name(w287) -> ("加标回收数据时间"=w290:timestamp, "加标回收实测值"=w289:sgl, "加标回收数据标识"=w288:string)
      }
      frame 8 {
        n144 = Unbundle By Name(w294) -> ("空白数据时间"=w293:timestamp, "空白实测值"=w292:sgl, "空白数据标识"=w291:string)
      }
      frame 9 {
        n145 = Unbundle By Name(w298) -> ("标样数据时间"=w297:timestamp, "标样实测值"=w296:sgl, "标样数据标识"=w295:string)
      }
      frame 10 {
        n146 = Unbundle By Name(w299) -> ("水样数据时间"=w302:timestamp, "水样实测值"=w301:sgl, "水样数据标识"=w300:string)
      }
    }
    n147 = Unbundle By Name(w223) -> ("因子编码"=w201:u32, "单位"=w198:u16)
    n148 = Not Equal To 0?(x=w198) -> (x != 0?=w199:bool)
    n149 = case shown="假" w199 {
      tunnel: ["mg/L" ("RingText.Text") w232] -> w203
      tunnel: w198 -> [_ w231]
      frame False {
      }
      frame True {
        n150 = property on="单位:" class="Enum (严格)"("Value"=w231) -> (error out=w233:errorcluster)  [unwired: 2 in, 1 out]
        n151 = property on="单位:" class="Enum (严格)"(error in=w233) -> ("RingText.Text"=w232:string)  [unwired: 1 in, 2 out]
      }
    }
    n152 = case shown="0" w221 {
      selector: w221 -> [w237 _ _ _ _ _ _ _ _ _ _ _ _ _ _ _]
      tunnel: [w238 "空闲" ("工作状态") "水样测量" ("工作状态") "标样核查" ("工作状态") "零点核查" ("工作状态") "跨度核查" ("工作状态") "空白测试" ("工作状态") "平行样测试" ("工作状态") "加标回收" ("工作状态") "空白校准" ("工作状态") "标样校准" ("工作状态") "初始化" ("工作状态") "调试" ("工作状态") "填充管路" ("工作状态") "清洗管路" ("工作状态") "清洗反应杯" ("工作状态")] -> w220
      frame Default {
        n153 = Format Into String(format string="%d" ("格式字符串"), initial string="未知" ("工作状态"), w237) -> (resulting string=w238:string)  [unwired: 1 in, 1 out]
      }
      frame 0 {
      }
      frame 1 {
      }
      frame 2 {
      }
      frame 3 {
      }
      frame 4 {
      }
      frame 5 {
      }
      frame 6 {
      }
      frame 7 {
      }
      frame 8 {
      }
      frame 9 {
      }
      frame 10 {
      }
      frame 22 {
      }
      frame 30 {
      }
      frame 31 {
      }
      frame 32 {
      }
    }
    n154 = case shown="默认" w219 {
      tunnel: ["" ("字符串") "低量程" ("字符串") "高量程" ("字符串")] -> w218
      frame Default {
      }
      frame 0 {
      }
      frame 1 {
      }
    }
    n155 = Format Into String(format string="w%05d" ("格式字符串"), w201) -> (resulting string=w200:string)  [unwired: 2 in, 1 out]
    n156 = Number To Fractional String(number=w209, precision (6)=i16 2 ("精度(6)")) -> (F-format string=w212:string)  [unwired: 2 in]
    n157 = Concatenate Strings(w212, " " ("字符串"), w203) -> (w210:string)
    n158 = call "告警码字段定义.vi"("告警代码"=w207) -> ("字符串"=w206:string)  [unwired: 8 in, 2 out]
    n159 = call "故障码字段定义.vi"("故障代码"=w205) -> ("字符串"=w204:string)  [unwired: 10 in]
    n160 = global read "VARCODMn全局变量.vi" "序列号"() -> (w222:string)
    n161 = Bundle By Name(cluster=T3 {"仪器编号:"="", "工作状态:"="", "运行量程: "="", "数据时间:"=timestamp(0 s since 1904-01-01), "实测值:"="", "数据标识: "="", "仪器时间:"=timestamp(0 s since 1904-01-01), "告警状态: "="", "故障状态:  "="", "因子编码:"=""} ("运行状态"), "仪器编号:"=w222, "工作状态:"=w220, "运行量程:"=w218, "仪器时间:"=w217, "数据时间:"=w214, "实测值:"=w210, "数据标识:"=w208, "告警状态:"=w206, "故障状态:"=w204, "因子编码:"=w200) -> (→"运行状态":T3)
  }
  n162 = while {
    tunnel: w52 -> [_]
    tunnel: w42 -> [w341]
    stop <- FALSE stop-if-true
    # "时序问题会缺少日志"
    n163 = global read "VARCODMn全局变量.vi" "状态告警区"() -> (w378:T18)
    n164 = global read "VARCODMn全局变量.vi" "状态告警区"() -> (w344:T18)
    n165 = global read "VARCODMn全局变量.vi" "状态告警区"() -> (w365:T18)
    n166 = global read "VARCODMn全局变量.vi" "状态告警区"() -> (w369:T18)
    n167 = Wait (ms)(milliseconds to wait=u32 1000 ("等待时间（毫秒）")) -> ()  [unwired: 1 out]
    n168 = global read "VARCODMn全局变量.vi" "状态告警区"() -> (w363:T18)
    n169 = Unbundle By Name(w378) -> ("id"=w375:u16, "flowid"=w377:u16, "量程"=w376:u16, "工作状态"=w355:u16, "A"=→"A":sgl, "B"=→"B":sgl, "K"=→"K":sgl, "当前滴定数"=→"当前滴定数":sgl, "T"=→"环境温度":sgl, "H"=→"环境湿度":sgl, "运行时间"=→"运行时间":sgl, "当前ORP值"=→"ORP值/光值":sgl, "加热实时温度"=w315:sgl, "当前步骤剩余时间"=→"当前步骤剩余时间":sgl, "结束滴定数"=→"终点滴定数":sgl, "注射泵保温温度"=→"注射泵保温温度":sgl, "匹配滴定数X0"=→"X0":u16)
    "加热实时温度" <- w315
    n170 = Unbundle By Name(w344) -> ("日志代码"=w360:u16)
    n171 = Unbundle By Name(w365) -> ("工作状态"=w348:u16, "id"=w347:u16)
    n172 = Unbundle By Name(w369) -> ("id"=w368:u16, "故障代码"=w327:u16, "告警代码"=w326:u16)
    n173 = Unbundle By Name(w363) -> ("日志代码"=w321:u16)
    n174 = local read "总步数"() -> (w320:i32)
    n175 = property on="多列列表框" class="MCListbox (严格)"() -> ("ItemNames"=w339:string[][])  [unwired: 2 in, 2 out]
    n176 = feedback-in #2(w360) -> ()
    n177 = feedback #2(w360) -> (w383:u16)
    n178 = feedback #3(w327) -> (w366:u16)
    n179 = feedback-in #3(w327) -> ()
    n180 = feedback #4(w326) -> (w343:u16)
    n181 = feedback-in #4(w326) -> ()
    n182 = Not Equal To 0?(x=w348) -> (x != 0?=w350:bool)
    n183 = Bundle("id"=w375, "flowid"=w377, "量程"=w376) -> (w370:cluster{"id":u16, "flowid":u16, "量程":u16})  [unwired: 1 in]
    n184 = call "消解压力计算.vi"("当前消解温度"=w315) -> ("消解压力"=→"消解压力kPa":dbl)  [unwired: 10 in]
    n185 = Not Equal To 0?(x=w355) -> (x != 0?=w380:bool)
    n186 = Subtract(x=w360, y=1) -> (x-y=→"多列列表框":i32)
    n187 = Divide(x=w321, y=w320) -> (x/y=w323:dbl)
    n188 = Empty Array?(array=w339) -> (empty?=w338:bool)
    n189 = call <vilib>:"Boolean Crossing PtByPt.vi"("direction"=enum16{"either", "false-true", "true-false"}."either", "input"=w380) -> ("crossing"=w354:bool)  [unwired: 1 in]
    n190 = Not Equal?(x=w360, y=w383) -> (x != y?=w382:bool)
    n191 = Not Equal?(x=w366, y=w327) -> (x != y?=w367:bool)
    n192 = Not Equal?(x=w343, y=w326) -> (x != y?=w342:bool)
    n193 = call <vilib>:"Boolean Crossing PtByPt.vi"("direction"=enum16{"either", "false-true", "true-false"}."false-true", "input"=w350) -> ("crossing"=w352:bool)  [unwired: 1 in]
    n194 = call <vilib>:"Boolean Crossing PtByPt.vi"("direction"=enum16{"either", "false-true", "true-false"}."true-false", "input"=w350) -> ("crossing"=w349:bool)  [unwired: 1 in]
    n195 = feedback #5(w321) -> (w364:u16)
    n196 = feedback-in #5(w321) -> ()
    n197 = Multiply(x=w323, y=100.0) -> (x*y=→"滑动杆":dbl)
    n198 = First Call?() -> (First Call?: T/F=w381:bool)
    n199 = Compound Arithmetic op=OR ("复合运算")(w354, w381, w338) -> (w379:bool)
    n200 = Not Equal?(x=w321, y=w364) -> (x != y?=w362:bool)
    n201 = case shown="真" w382 {
      tunnel: w360 -> [_ w539]
      frame False {
      }
      frame True {
        n202 = Subtract(x=w539, y=1) -> (x-y=w537:i32)
        n203 = Subtract(x=w537, y=5) -> (x-y=w541:i32)
        n204 = Greater Or Equal To 0?(x=w541) -> (x >= 0?=w540:bool)
        n205 = property on="多列列表框" class="MCListbox (严格)"() -> (error out=w545:errorcluster, "TopLeft"=w546:T22)  [unwired: 2 in, 1 out]
        n206 = Select(t=w541, s=w540, f=0) -> (s? t:f=w542:i32)
        n207 = Bundle By Name(cluster=w546, "Row"=w542) -> (w547:T22)
        n208 = property on="多列列表框" class="MCListbox (严格)"(error in=w545, "TopLeft"=w547) -> ()  [unwired: 1 in, 2 out]
      }
    }
    n209 = case shown="真" w352 {
      tunnel: w347 -> [_ w408]
      tunnel: w348 -> [_ w413]
      frame False {
      }
      frame True {
        n210 = case shown="8" w413 {
          tunnel: [_ "【水样测试】" ("字符串") "【标样核查】" ("字符串") "【零点核查】" ("字符串") "【跨度核查】" ("字符串") "【空白测试】" ("字符串") "【平行样测试】" ("字符串") "【加标回收】" ("字符串") "【空白校准】" ("字符串") "【标样校准】" ("字符串")] -> w412
          frame 0, Default {
          }
          frame 1 {
          }
          frame 2 {
          }
          frame 3 {
          }
          frame 4 {
          }
          frame 5 {
          }
          frame 6 {
          }
          frame 7 {
          }
          frame 8 {
          }
          frame 9 {
          }
        }
        n211 = call "id参数转换.vi"("id"=w408) -> ("table输出"=w407:string)  [unwired: 10 in]
        n212 = Concatenate Strings("<<" ("字符串"), w412, "启动" ("字符串")) -> (w411:string)
        n213 = Get Date/Time In Seconds() -> (seconds since 1Jan1904=w415:timestamp)
        n214 = Bundle By Name(cluster=T20 {"时间标识"=timestamp(0 s since 1904-01-01), "设备"="", "日志信息"="", "流程参数"=""} ("data in"), "时间标识"=w415, "设备"=w407, "日志信息"=w411) -> (w414:T20)
        n215 = call "CODMn操作日志.vi"("data in"=w414) -> ()  [unwired: 11 in]
      }
    }
    n216 = case shown="真" w349 {
      tunnel: w347 -> [_ w390]
      tunnel: w348 -> [_ w394]
      frame False {
      }
      frame True {
        n217 = case shown="1" w394 {
          tunnel: [_ "【水样测试】" ("字符串") "【标样核查】" ("字符串") "【零点核查】" ("字符串") "【跨度核查】" ("字符串") "【空白测试】" ("字符串") "【平行样测试】" ("字符串") "【加标回收】" ("字符串") "【空白校准】" ("字符串") "【标样校准】" ("字符串")] -> w393
          frame 0, Default {
          }
          frame 1 {
          }
          frame 2 {
          }
          frame 3 {
          }
          frame 4 {
          }
          frame 5 {
          }
          frame 6 {
          }
          frame 7 {
          }
          frame 8 {
          }
          frame 9 {
          }
        }
        n218 = call "id参数转换.vi"("id"=w390) -> ("table输出"=w389:string)  [unwired: 10 in]
        n219 = Concatenate Strings(w393, "停止" ("字符串"), ">>" ("字符串")) -> (w392:string)
        n220 = Get Date/Time In Seconds() -> (seconds since 1Jan1904=w396:timestamp)
        n221 = Bundle By Name(cluster=T20 {"时间标识"=timestamp(0 s since 1904-01-01), "设备"="", "日志信息"="", "流程参数"=""} ("data in"), "时间标识"=w396, "设备"=w389, "日志信息"=w392) -> (w395:T20)
        n222 = call "CODMn操作日志.vi"("data in"=w395) -> ()  [unwired: 11 in]
      }
    }
    n223 = case shown="0" w348 {
      frame 0 {
        n224 = local write "数组"(string[] [] ("数组")) -> ()
      }
      frame 1, Default {
      }
    }
    n225 = case shown="真" w362 {
      frame False {
      }
      frame True {
        n226 = property on="多列列表框" class="MCListbox (严格)"() -> ("ItemNames"=w430:string[][], "Value"=w431:i32)  [unwired: 2 in, 2 out]
        n227 = Index Array(array=w430, index (row)=w431) -> (element=w429:string[])  [unwired: 1 in]
        n228 = Index Array(array=w429) -> (element=w428:string)  [unwired: 1 in]
        n229 = call "过滤筛选流程.vi"("字符串"=w428) -> ("匹配后偏移量"=w427:i32)  [unwired: 10 in]
        n230 = case shown="默认" w427 {
          tunnel: w428 -> [_ w432]
          frame -1 {
          }
          frame Default {
            # "步骤日志存储"
            n231 = case shown="默认" w432 {
              selector: w432 -> [w438 w440]
              tunnel: [w438 w440] -> w434
              tunnel: [string[] [] ("数组") "数组"] -> w433
              frame "读数" {
              }
              frame Default {
              }
            }
            n232 = for {
              N: 1 -> [_]
              tunnel: w434 -> [w442]
              shift-right: [w441] -> w435
              shift-left: w433 -> [w443]
              n233 = Search 1D Array(1D array=w443, element=w442) -> (index of element=w446:i32)  [unwired: 1 in]
              n234 = Format Into String(format string="%s" ("格式字符串"), w442) -> (resulting string=w447:string)  [unwired: 2 in, 1 out]
              n235 = Equal?(x=w446, y=-1) -> (x = y?=w444:bool)
              n236 = case shown="真" w444 {
                tunnel: w447 -> [_ w455]
                tunnel: w443 -> [w449 w459]
                tunnel: w442 -> [_ w458]
                tunnel: [w449 w457] -> w441
                frame False {
                }
                frame True {
                  n237 = Insert Into Array(array=w459, new element=w458) -> (w457:string[])  [unwired: 1 in]
                  n238 = case shown="\"初始化\"" w455 {
                    selector: w455 -> [w484 w487 w490]
                    tunnel: [w484 w486 w489] -> w451
                    frame Default {
                    }
                    frame "初始化" {
                      n239 = Concatenate Strings("<<" ("字符串"), w487) -> (w486:string)
                    }
                    frame "结束" {
                      n240 = Concatenate Strings(w490, ">>" ("字符串")) -> (w489:string)
                    }
                  }
                  n241 = global read "VARCODMn全局变量.vi" "状态告警区"() -> (w454:T18)
                  n242 = Unbundle By Name(w454) -> ("工作状态"=w453:u16)
                  n243 = global read "VARCODMn全局变量.vi" "状态告警区"() -> (w474:T18)
                  n244 = case shown="1" w453 {
                    tunnel: [_ "【水样测试】" ("字符串") "【标样核查】" ("字符串") "【零点核查】" ("字符串") "【跨度核查】" ("字符串") "【空白测试】" ("字符串") "【平行样测试】" ("字符串") "【加标回收】" ("字符串") "【空白校准】" ("字符串") "【标样校准】" ("字符串")] -> w452
                    frame 0, Default {
                    }
                    frame 1 {
                    }
                    frame 2 {
                    }
                    frame 3 {
                    }
                    frame 4 {
                    }
                    frame 5 {
                    }
                    frame 6 {
                    }
                    frame 7 {
                    }
                    frame 8 {
                    }
                    frame 9 {
                    }
                  }
                  n245 = global read "VARCODMn全局变量.vi" "状态告警区"() -> (w469:T18)
                  n246 = Unbundle By Name(w474) -> ("id"=w473:u16)
                  n247 = case shown="1, 21, 131" w473 {
                    tunnel: [_ "CODMn" ("table输入") "氨氮" ("table输入") "总氮" ("table输入")] -> w471
                    frame Default {
                    }
                    frame 1, 21, 131 {
                    }
                    frame 3, 92 {
                    }
                    frame 2, 76 {
                    }
                  }
                  n248 = Unbundle By Name(w469) -> ("A"=w466:sgl, "B"=w465:sgl, "K"=w464:sgl, "当前滴定数"=w463:sgl, "id"=w462:u16, "flowid"=w461:u16, "量程"=w460:u16)
                  n249 = Concatenate Strings(w452, w451) -> (w450:string)
                  n250 = Format Into String(format string="A=%#f,B=%#f,K=%#f,当前滴定数=%#f,Flow=%d-%-d-%-d" ("格式字符串"), w466, w465, w464, w463, w462, w461, w460) -> (resulting string=w467:string)  [unwired: 2 in, 1 out]
                  n251 = Get Date/Time In Seconds() -> (seconds since 1Jan1904=w470:timestamp)
                  n252 = Bundle By Name(cluster=T20 {"时间标识"=timestamp(0 s since 1904-01-01), "设备"="", "日志信息"="", "流程参数"=""} ("data in"), "时间标识"=w470, "设备"=w471, "日志信息"=w450, "流程参数"=w467) -> (w472:T20)
                  n253 = call "CODMn操作日志.vi"("data in"=w472) -> ()  [unwired: 11 in]
                }
              }
            }
            n254 = local write "数组"(w435) -> ()
          }
        }
      }
    }
    n255 = Not Equal To 0?(x=w326) -> (x != 0?=w328:bool)
    n256 = Not Equal To 0?(x=w327) -> (x != 0?=w329:bool)
    n257 = Or(x=w329, y=w328) -> (x .or. y?=w325:bool)
    n258 = case shown="真" w325 {
      tunnel: w368 -> [_ w500]
      tunnel: w367 -> [_ w499]
      tunnel: w342 -> [_ w497]
      tunnel: w326 -> [_ w496]
      tunnel: w341 -> [_ w495]
      tunnel: w327 -> [_ w494]
      frame False {
      }
      frame True {
        n259 = Or(x=w497, y=w499) -> (x .or. y?=w498:bool)
        n260 = case shown="真" w498 {
          tunnel: w500 -> [_ w515]
          tunnel: w494 -> [_ w507]
          tunnel: w496 -> [_ w506]
          tunnel: w495 -> [_ w505]
          frame False {
          }
          frame True {
            n261 = call "故障码字段定义.vi"("故障代码"=w507) -> ("字符串"=w503:string)  [unwired: 10 in]
            n262 = call "告警码字段定义.vi"("告警代码"=w506) -> ("故障详情"=w501:string, "通用告警信息"=w502:string)  [unwired: 8 in, 1 out]
            n263 = Format Into String(format string="【%s】%s" ("格式字符串"), initial string="" ("初始字符串"), w503, w502) -> (resulting string=w512:string)  [unwired: 1 in, 1 out]
            n264 = call "id参数转换.vi"("id"=w515) -> ("table输出"=w504:string)  [unwired: 10 in]
            n265 = Search and Replace String(replace all?=TRUE ("替换全部？(F)"), input string=w512, search string="【无故障】|无告警" ("字符串")) -> (result string=w509:string)  [unwired: 5 in, 3 out]
            n266 = call "balloon入队列.vi"("队列"=w505, "故障详情"=w501, "告警信息"=w502, "故障信息"=w503, "参数名称"=w504) -> ()  [unwired: 6 in, 1 out]
            n267 = Get Date/Time In Seconds() -> (seconds since 1Jan1904=w516:timestamp)
            n268 = Bundle By Name(cluster=T21 {"时间标识"=timestamp(0 s since 1904-01-01), "设备"="", "日志信息"="", "备注"=""} ("data in"), "时间标识"=w516, "设备"=w504, "日志信息"=w509, "备注"=w501) -> (w517:T21)
            n269 = call "CODMn报警信息.vi"("data in"=w517) -> ()  [unwired: 10 in, 1 out]
          }
        }
      }
    }
    n270 = while {
      tunnel: w379 -> [w525]
      tunnel: w370 -> [w524]
      shift-right: [w521] -> _
      shift-left: _ -> [w522]
      shift-right: [w518] -> _
      shift-left: _ -> [w520]
      stop <- TRUE stop-if-true
      # "XML解析步骤显示"
      n271 = case shown="真" w525 {
        tunnel: [w527 w535] -> w518
        tunnel: [w526 w534] -> w521
        tunnel: w524 -> [_ w529]
        tunnel: w520 -> [w527 _]
        tunnel: w522 -> [w526 _]
        frame False {
        }
        frame True {
          n272 = call "斯坦道XML解析.vi"("添加的路径"="流程路径", "参数簇"=w529) -> ("步骤时间"=w530:string[], "步骤名"=w532:string[])  [unwired: 8 in]
          n273 = for {
            tunnel: w532 -> [_] mode=indexing
            tunnel: [w536] -> w533 mode=indexing
            i -> [w536]
          }
          n274 = Build Array(w532, w530) -> (w531:string[][])
          n275 = Transpose 2D Array(2D array=w531) -> (transposed array=w534:string[][])
          n276 = Number To Decimal String(number=w533) -> (decimal integer string=w535:string[])  [unwired: 1 in]
        }
      }
      n277 = Array Size(array=w518) -> (size(s)=→"总步数":i32)
      n278 = property on="多列列表框" class="MCListbox (严格)"("ItemNames"=w521, "RowHdrs[]"=w518) -> ()  [unwired: 2 in, 2 out]
    }
    n279 = global read "VARCODMn全局变量.vi" "ORP滴定曲线"() -> (→"ORP滴定曲线":u16[])
    n280 = global read "VARCODMn全局变量.vi" "滴定数-ORP值"() -> (→"滴定数-ORP值":u16[])
    n281 = global read "VARCODMn全局变量.vi" "波形时间"() -> (→"波形时间":timestamp)
    n282 = global read "VARCODMn全局变量.vi" "页面"() -> (w318:enum16{"主页", "参数页", "校准页"})
    n283 = case shown="\"参数页\"" w318 {
      tunnel: [_ _ TRUE ("可见")] -> w317
      tunnel: [_ TRUE ("可见") _] -> w316
      frame "主页", Default {
      }
      frame "参数页" {
      }
      frame "校准页" {
      }
    }
    n284 = global read "VARCODMn全局变量.vi" "温度波形时间"() -> (→"温度波形时间":timestamp)
    n285 = global read "VARCODMn全局变量.vi" "时间-温度"() -> (→"时间-温度":u16[])
    n286 = global read "VARCODMn全局变量.vi" "温度曲线"() -> (→"ORP滴定曲线 2":u16[])
    n287 = property on="参数查询" class="Bool"("Visible"=w317) -> ()  [unwired: 2 in, 2 out]
    n288 = property on="仪器校准" class="Bool"("Visible"=w316) -> ()  [unwired: 2 in, 2 out]
  }
  n289 = control-ref of="测量模式下拉列表"() -> (w54:refnum<vi>)
  n290 = control-ref of="校准按钮"() -> (w24:refnum<vi>)
  n291 = control-ref of="参数下拉列表"() -> (w55:refnum<vi>)
  n292 = control-ref of="量程下拉列表"() -> (w56:refnum<vi>)
  n293 = control-ref of="校准按钮"() -> (w45:refnum<vi>)
  n294 = control-ref of="曲线模型"() -> (w44:refnum<vi>)
  n295 = control-ref of="公式"() -> (w53:refnum<vi>)
  n296 = while {
    tunnel: w46 -> [w551]
    tunnel: w24 -> [w549]
    tunnel: w23 -> [w548]
    tunnel: w20 -> [_]
    tunnel: w12 -> [_]
    stop <- FALSE stop-if-true
    n297 = event shown="[4] \"校准按钮.校准1\", \"校准按钮.校准2\", \"校准按钮.校准3\", \"校准按钮.校准4\", \"校准按钮.校准5\": 鼠标按下" {
      selector: _ -> [_ _ _ _ _ _ _]
      dyn-events: _ -> [_ _ _ _ _ _ _]
      timeout: _ -> [_ _ _ _ _ _ _]
      tunnel: [_ _ _ w576 w633 w797 w839] -> w550
      tunnel: w548 -> [_ _ _ w575 w636 w808 w835]
      tunnel: w549 -> [_ _ _ _ w635 w812 _]
      tunnel: w551 -> [_ _ _ _ w634 _ _]
      event Timeout {
        # "始终在超时后终止\n事件结构。在事件结构的其它情况下决不终止循环。"
        n298 = event-data() -> ()  [unwired: 1 in, 2 out]
      }
      event "曲线模型.标液浓度1", "曲线模型.标液浓度2", "曲线模型.标液浓度3", "曲线模型.标液浓度4", "曲线模型.标液浓度5", "曲线模型.精度": Mouse Down {
        n299 = event-data() -> ("CtlRef"=w557:refnum<vi>)  [unwired: 1 in, 7 out]
        n300 = property class="DigNum (严格)"(reference=w557) -> (reference out=w556:refnum<vi>, "Value"=w553:dbl)  [unwired: 1 in, 1 out]
        n301 = call "数字键盘.vi"("OldNumber"=w553) -> ("NewNumber"=w554:dbl)
        n302 = Equal?(x=w553, y=w554) -> (x = y?=w555:bool)
        n303 = case shown="假" w555 {
          tunnel: w556 -> [w559 _]
          tunnel: w554 -> [w558 _]
          frame False {
            n304 = property class="DigNum (严格)"(reference=w559, "Val(Sgnl)"=w558) -> ()  [unwired: 1 in, 2 out]
          }
          frame True {
          }
        }
      }
      event "曲线模型.测量吸光度1", "曲线模型.测量吸光度2", "曲线模型.测量吸光度3", "曲线模型.测量吸光度4", "曲线模型.测量吸光度5": Mouse Down {
        n305 = event-data() -> ("CtlRef"=w563:refnum<vi>)  [unwired: 1 in, 7 out]
        n306 = property class="DigNum (严格)"(reference=w563) -> (reference out=w562:refnum<vi>, "Value"=w561:dbl)  [unwired: 1 in, 1 out]
        n307 = call "数字键盘.vi"("OldNumber"=w561) -> ("NewNumber"=w560:dbl)
        n308 = property class="DigNum (严格)"(reference=w562, "Val(Sgnl)"=w560) -> ()  [unwired: 1 in, 2 out]
      }
      event "曲线模型.标液浓度1", "曲线模型.测量吸光度1", "曲线模型.标液浓度2", "曲线模型.测量吸光度2", "曲线模型.样品1启用", "曲线模型.样品2启用", "曲线模型.标液浓度3", "曲线模型.测量吸光度3", "曲线模型.样品3启用", "曲线模型.标液浓度4", "曲线模型.测量吸光度4", "曲线模型.样品4启用", "曲线模型.标液浓度5", "曲线模型.测量吸光度5", "曲线模型.样品5启用", "曲线模型.模型", "曲线模型.method", "曲线模型.精度": Value Change {
        n309 = event-data() -> ()  [unwired: 1 in, 6 out]
        n310 = property class="Clust (严格)"(reference=w575) -> ("Value"=w574:T5)  [unwired: 1 in, 2 out]
        n311 = call <vilib>:"Application Directory.vi"() -> ("Application Directory"=w595:path)
        n312 = Build Path(base path=w595, name or relative path="config" ("名称或相对路径")) -> (appended path=w593:path)
        n313 = Unbundle By Name(w574) -> ("模型"=w619:enum32{"线性", "多项式"}, "标液浓度1"=w615:dbl, "标液浓度2"=w614:dbl, "标液浓度3"=w613:dbl, "标液浓度4"=w612:dbl, "标液浓度5"=w611:dbl, "测量吸光度1"=w608:dbl, "测量吸光度2"=w607:dbl, "测量吸光度3"=w606:dbl, "测量吸光度4"=w605:dbl, "测量吸光度5"=w604:dbl, "样品1启用"=w602:bool, "样品2启用"=w601:bool, "样品3启用"=w600:bool, "样品4启用"=w599:bool, "样品5启用"=w598:bool, "method"=w618:enum16{"最小二乘", "最小绝对残差", "Bisquare"}, "精度"=w617:dbl)
        n314 = call <vilib>:"Check if File or Folder Exists.vi"("path"=w593) -> ("file or folder exists?"=w592:bool, "dup path"=w591:path)  [unwired: 8 in, 1 out]
        n315 = case shown="真" w592 {
          tunnel: w591 -> [w629 w630]
          tunnel: [w628 w630] -> w588
          frame False {
            n316 = Create Folder(path (use dialog)=w629) -> (created path=w628:path)  [unwired: 2 in, 2 out]
          }
          frame True {
          }
        }
        n317 = Insert Into Array(array=dbl[] [] ("标液浓度"), new element #1=w615, new element #2=w614, new element #3=w613, new element #4=w612, new element #5=w611) -> (w610:dbl[])  [unwired: 1 in]
        n318 = Insert Into Array(array=dbl[] [] ("标液浓度"), new element #1=w608, new element #2=w607, new element #3=w606, new element #4=w605, new element #5=w604) -> (w567:dbl[])  [unwired: 1 in]
        n319 = Insert Into Array(array=bool[] [] ("启用"), new element #1=w602, new element #2=w601, new element #3=w600, new element #4=w599, new element #5=w598) -> (w568:bool[])  [unwired: 1 in]
        n320 = for {
          tunnel: w568 -> [w623] mode=indexing
          tunnel: w567 -> [w622] mode=indexing
          shift-right: [w620] -> w565
          shift-left: dbl[] [] -> [w621]
          n321 = case shown="真" w623 {
            tunnel: w622 -> [_ w627]
            tunnel: w621 -> [w624 w626]
            tunnel: [w624 w625] -> w620
            frame False {
            }
            frame True {
              n322 = Build Array (concatenate)(w626, w627) -> (w625:dbl[])
            }
          }
        }
        n323 = Concatenate Strings("曲线模型" ("字符串"), ".ini" ("字符串")) -> (w590:string)
        n324 = call "CODMn线性公式.vi"("标液浓度"=w610, "信号值"=w567, "启用"=w568, "method"=w618, "模型"=w619, "精度"=w617) -> ("拟合方程"=w597:string, "r^2"=w571:dbl, "XY图"=w596:cluster{"X Values":dbl[], "Y Values":dbl[]}[], "Polynomial Coefficients"=w572:dbl[])  [unwired: 7 in, 3 out]
        n325 = Bundle By Name(cluster=w574, "拟合公式"=w597, "r^2"=w571, "XY图"=w596) -> (w573:T5)
        n326 = local write "曲线模型"(w573) -> ()
        n327 = Array Max & Min(array=w565) -> (max value=w564:dbl)  [unwired: 3 out]
        n328 = Bundle By Name(cluster=T10 {"曲线模型"={"标液浓度1"=0.0, "测量吸光度1"=0.0, "样品1启用"=FALSE, "标液浓度2"=0.0, "测量吸光度2"=0.0, "样品2启用"=FALSE, "标液浓度3"=0.0, "测量吸光度3"=0.0, "样品3启用"=FALSE, "标液浓度4"=0.0, "测量吸光度4"=0.0, "样品4启用"=FALSE, "标液浓度5"=0.0, "测量吸光度5"=0.0, "样品5启用"=FALSE, "模型"=enum."线性", "method"=enum."最小二乘", "精度"=7.0, "XY图"=[], "拟合公式"="", "r^2"=0.0, "零点校准时间"=timestamp(0 s since 1904-01-01), "标液校准时间1"=timestamp(0 s since 1904-01-01), "标液校准时间2"=timestamp(0 s since 1904-01-01), "标液校准时间3"=timestamp(0 s since 1904-01-01), "标液校准时间4"=timestamp(0 s since 1904-01-01)}, "Polynomial Coefficients"=[]} ("输出簇"), "曲线模型"=w573, "Polynomial Coefficients"=w572) -> (w580:T10)
        n329 = Build Path(base path=w588, name or relative path=w590) -> (appended path=w581:path)
        n330 = Array To Cluster(array=w572) -> (cluster=w570:T16)
        n331 = local read "模型选择"() -> (w579:cluster{"参数":u8, "测量模式":u8, "量程":u8})
        n332 = local write "公式切换阈值滴定数(0~9999)"(w564) -> ()
        n333 = local write "公式"(w570) -> ()
        n334 = Flatten To String(anything=w579) -> (data string=w587:string)  [unwired: 3 in, 2 out]
        n335 = call <vilib>:"Open Config Data.vi"("configuration file path"=w581) -> ("error out"=w584:errorcluster, "refnum"=w585:T12)  [unwired: 8 in, 1 out]
        n336 = local read "公式、校准输出"() -> (w578:T6)
        n337 = call <userlib>:"Write Section Cluster__ogtk.vi"("section (optional)"=w587, "error in (no error)"=w584, "Section Formatted Cluster"=w580, "refnum"=w585) -> ("error out"=w582:errorcluster, "dup refnum"=w583:T12)  [unwired: 6 in]
        n338 = Bundle By Name(cluster=w578, "公式"=w570, "校准.校准？"=FALSE) -> (w576:T6)
        n339 = call <vilib>:"Close Config Data.vi"("error in (no error)"=w582, "refnum"=w583) -> ()  [unwired: 8 in, 2 out]
        n340 = global write "CODMn断电保存全局变量.vi" "公式、校准输出"(w576) -> ()
      }
      event "校准按钮.校准1", "校准按钮.校准2", "校准按钮.校准3", "校准按钮.校准4", "校准按钮.校准5": Mouse Down {
        n341 = event-data() -> ("CtlRef"=w637:refnum<vi>)  [unwired: 1 in, 7 out]
        n342 = property class="Bool (严格)"(reference=w637) -> ("Label.Text"=w632:string)  [unwired: 1 in, 2 out]
        n343 = case shown="\"校准1\"" w632 {
          tunnel: [FALSE ("T button?") w639 w643 w647 w651 w655] -> w631
          frame "假", Default {
          }
          frame "校准1" {
            n344 = Two Button Dialog(message="是否选择数据表中已有的空白校准数据" ("消息"), 1:"否" ("F按钮名称（“取消”）"), 2:"是" ("T按钮名称（“确定”）")) -> (T button?=w639:bool)
          }
          frame "校准2" {
            n345 = Two Button Dialog(message="是否选择数据表中已有的标样校准数据" ("消息"), 1:"否" ("F按钮名称（“取消”）"), 2:"是" ("T按钮名称（“确定”）")) -> (T button?=w643:bool)
          }
          frame "校准3" {
            n346 = Two Button Dialog(message="是否选择数据表中已有的标样核查数据" ("消息"), 1:"否" ("F按钮名称（“取消”）"), 2:"是" ("T按钮名称（“确定”）")) -> (T button?=w647:bool)
          }
          frame "校准4" {
            n347 = Two Button Dialog(message="是否选择数据表中已有的零点核查数据" ("消息"), 1:"否" ("F按钮名称（“取消”）"), 2:"是" ("T按钮名称（“确定”）")) -> (T button?=w651:bool)
          }
          frame "校准5" {
            n348 = Two Button Dialog(message="是否选择数据表中已有的跨度核查数据" ("消息"), 1:"否" ("F按钮名称（“取消”）"), 2:"是" ("T按钮名称（“确定”）")) -> (T button?=w655:bool)
          }
        }
        n349 = case shown="真" w631 {
          tunnel: w632 -> [w671 w704]
          tunnel: w636 -> [w667 w703]
          tunnel: w635 -> [w666 _]
          tunnel: w634 -> [w662 _]
          tunnel: [w661 w705] -> w633
          frame False {
            w665 = T23."Disabled and Grayed Out" ("禁用")
            n350 = case shown="\"校准5\"" w671 {
              tunnel: [w693 w694 w697 w698 w700] -> w669
              tunnel: [u16 1 ("校准点1-5") u16 2 ("校准点1-5") u16 3 ("校准点1-5") u16 4 ("校准点1-5") u16 5 ("校准点1-5")] -> w659
              frame "校准1", Default {
                n351 = control-ref of="标液浓度1"() -> (w693:refnum<vi>)
              }
              frame "校准2" {
                n352 = control-ref of="标液浓度2"() -> (w694:refnum<vi>)
              }
              frame "校准3" {
                n353 = control-ref of="标液浓度3"() -> (w697:refnum<vi>)
              }
              frame "校准4" {
                n354 = control-ref of="标液浓度4"() -> (w698:refnum<vi>)
              }
              frame "校准5" {
                n355 = control-ref of="标液浓度5"() -> (w700:refnum<vi>)
              }
            }
            n356 = property class="DigNum (严格)"(reference=w669) -> ("Value"=w664:dbl)  [unwired: 1 in, 2 out]
            n357 = local read "量程下拉列表"() -> (w660:enum16{"低量程1", "低量程2", "高量程1", "高量程2"})
            n358 = property class="Clust (严格)"(reference=w666, "DisabledEnum"=w665) -> ()  [unwired: 1 in, 2 out]
            n359 = property class="Clust (严格)"(reference=w667, "DisabledEnum"=w665) -> ()  [unwired: 1 in, 2 out]
            n360 = Equal To 0?(x=w664) -> ()  [unwired: 1 out]
            n361 = case shown="1" w659 {
              tunnel: [w672 w676 w680 w684 w689] -> w663
              tunnel: w660 -> [w673 w677 w681 w685 w688]
              frame 2, Default {
                # "校标"
                n362 = case shown="\"高量程1\"" w673 {
                  tunnel: [cluster{"命令":string, "data":variant} {"命令"="启动", "data"=variant(cluster{"站号":u16, "控制命令":u16[]} {"站号"=21, "控制命令"=[2304, 0]})} ("元素") cluster{"命令":string, "data":variant} {"命令"="启动", "data"=variant(cluster{"站号":u16, "控制命令":u16[]} {"站号"=21, "控制命令"=[2304, 256]})} ("元素")] -> w672
                  frame "低量程1", Default {
                  }
                  frame "高量程1" {
                  }
                }
              }
              frame 3 {
                # "标样核查"
                n363 = case shown="\"低量程1\", 默认" w677 {
                  tunnel: [w678 cluster{"命令":string, "data":variant} {"命令"="启动", "data"=variant(cluster{"站号":u16, "控制命令":u16[]} {"站号"=21, "控制命令"=[512, 256]})} ("元素")] -> w676
                  frame "低量程1", Default {
                    w678 = cluster{"命令":string, "data":variant} {"命令"="启动", "data"=variant(cluster{"站号":u16, "控制命令":u16[]} {"站号"=21, "控制命令"=[512, 0]})}  # 标样核查
                  }
                  frame "高量程1" {
                  }
                }
              }
              frame 4 {
                # "零点核查"
                n364 = case shown="\"高量程1\"" w681 {
                  tunnel: [w682 cluster{"命令":string, "data":variant} {"命令"="启动", "data"=variant(cluster{"站号":u16, "控制命令":u16[]} {"站号"=21, "控制命令"=[768, 256]})} ("元素")] -> w680
                  frame "低量程1", Default {
                    w682 = cluster{"命令":string, "data":variant} {"命令"="启动", "data"=variant(cluster{"站号":u16, "控制命令":u16[]} {"站号"=21, "控制命令"=[768, 0]})}  # 零点核查
                  }
                  frame "高量程1" {
                  }
                }
              }
              frame 5 {
                # "跨度核查"
                n365 = case shown="\"低量程1\", 默认" w685 {
                  tunnel: [w686 cluster{"命令":string, "data":variant} {"命令"="启动", "data"=variant(cluster{"站号":u16, "控制命令":u16[]} {"站号"=21, "控制命令"=[1024, 256]})} ("元素")] -> w684
                  frame "低量程1", Default {
                    w686 = cluster{"命令":string, "data":variant} {"命令"="启动", "data"=variant(cluster{"站号":u16, "控制命令":u16[]} {"站号"=21, "控制命令"=[1024, 0]})}  # 跨度核查
                  }
                  frame "高量程1" {
                  }
                }
              }
              frame 1 {
                # "校零"
                n366 = case shown="\"高量程1\"" w688 {
                  tunnel: [cluster{"命令":string, "data":variant} {"命令"="启动", "data"=variant(cluster{"站号":u16, "控制命令":u16[]} {"站号"=21, "控制命令"=[2048, 0]})} ("元素") cluster{"命令":string, "data":variant} {"命令"="启动", "data"=variant(cluster{"站号":u16, "控制命令":u16[]} {"站号"=21, "控制命令"=[2048, 256]})} ("元素")] -> w689
                  frame "低量程1", Default {
                  }
                  frame "高量程1" {
                  }
                }
              }
            }
            n367 = local read "公式、校准输出"() -> (w668:T6)
            n368 = Bundle By Name(cluster=w668, "校准.校准？"=TRUE ("校准？"), "校准.校准点1-5"=w659, "校准.校准浓度"=w664) -> (w661:T6)
            n369 = global write "CODMn断电保存全局变量.vi" "公式、校准输出"(w661) -> ()
            n370 = Enqueue Element(queue=w662, element=w663) -> ()  [unwired: 2 in, 3 out]
          }
          frame True {
            n371 = case shown="\"校准5\"" w704 {
              tunnel: w703 -> [_ w710 w728 w746 w764 w782]
              tunnel: "量程下拉列表 2" -> [_ w706 w724 w742 w760 w778]
              frame "假", Default {
              }
              frame "校准1" {
                n372 = property class="Clust (严格)"(reference=w710) -> ("Value"=w709:T5)  [unwired: 1 in, 2 out]
                n373 = call "校准数据选择表.vi"("量程下拉列表"=w706) -> ("布尔"=w707:bool, "ItemNames"=w708:string[])  [unwired: 9 in]
                n374 = case shown="真" w707 {
                  tunnel: w710 -> [_ w723]
                  tunnel: w709 -> [_ w722]
                  tunnel: w708 -> [_ w717]
                  frame False {
                  }
                  frame True {
                    n375 = Index Array(array=w717, index #2=7 ("索引"), index #3=11 ("索引")) -> (element #1=w714:string, element #2=w712:string, element #3=w713:string)  [unwired: 1 in]
                    n376 = Scan From String(format string="%<%Y/%m/%d %H:%M:%S>T" ("格式字符串"), input string=w714) -> (output 1=w719:timestamp)  [unwired: 3 in, 3 out]
                    n377 = Fract/Exp String To Number(string=w712) -> (number=w711:dbl)  [unwired: 3 in, 1 out]
                    n378 = Decimal String To Number(string=w713) -> (number=w718:i32)  [unwired: 2 in, 1 out]
                    n379 = Bundle By Name(cluster=w722, "标液浓度1"=w711, "测量吸光度1"=w718, "零点校准时间"=w719) -> (w721:T5)
                    n380 = property class="Clust (严格)"(reference=w723, "Val(Sgnl)"=w721) -> ()  [unwired: 1 in, 2 out]
                  }
                }
              }
              frame "校准2" {
                n381 = property class="Clust (严格)"(reference=w728) -> ("Value"=w727:T5)  [unwired: 1 in, 2 out]
                n382 = call "校准数据选择表.vi"("量程下拉列表"=w724) -> ("布尔"=w725:bool, "ItemNames"=w726:string[])  [unwired: 9 in]
                n383 = case shown="真" w725 {
                  tunnel: w728 -> [_ w741]
                  tunnel: w727 -> [_ w740]
                  tunnel: w726 -> [_ w735]
                  frame False {
                  }
                  frame True {
                    n384 = Index Array(array=w735, index #2=7 ("索引"), index #3=11 ("索引")) -> (element #1=w732:string, element #2=w730:string, element #3=w731:string)  [unwired: 1 in]
                    n385 = Scan From String(format string="%<%Y/%m/%d %H:%M:%S>T" ("格式字符串"), input string=w732) -> (output 1=w737:timestamp)  [unwired: 3 in, 3 out]
                    n386 = Fract/Exp String To Number(string=w730) -> (number=w729:dbl)  [unwired: 3 in, 1 out]
                    n387 = Decimal String To Number(string=w731) -> (number=w736:i32)  [unwired: 2 in, 1 out]
                    n388 = Bundle By Name(cluster=w740, "标液浓度2"=w729, "测量吸光度2"=w736, "标液校准时间1"=w737) -> (w739:T5)
                    n389 = property class="Clust (严格)"(reference=w741, "Val(Sgnl)"=w739) -> ()  [unwired: 1 in, 2 out]
                  }
                }
              }
              frame "校准3" {
                n390 = property class="Clust (严格)"(reference=w746) -> ("Value"=w745:T5)  [unwired: 1 in, 2 out]
                n391 = call "校准数据选择表.vi"("量程下拉列表"=w742) -> ("布尔"=w743:bool, "ItemNames"=w744:string[])  [unwired: 9 in]
                n392 = case shown="真" w743 {
                  tunnel: w746 -> [_ w759]
                  tunnel: w745 -> [_ w758]
                  tunnel: w744 -> [_ w750]
                  frame False {
                  }
                  frame True {
                    n393 = Index Array(array=w750, index #2=7 ("索引"), index #3=11 ("索引")) -> (element #1=w749:string, element #2=w748:string, element #3=w747:string)  [unwired: 1 in]
                    n394 = Scan From String(format string="%<%Y/%m/%d %H:%M:%S>T" ("格式字符串"), input string=w749) -> (output 1=w755:timestamp)  [unwired: 3 in, 3 out]
                    n395 = Fract/Exp String To Number(string=w748) -> (number=w754:dbl)  [unwired: 3 in, 1 out]
                    n396 = Decimal String To Number(string=w747) -> (number=w753:i32)  [unwired: 2 in, 1 out]
                    n397 = Bundle By Name(cluster=w758, "标液浓度3"=w754, "测量吸光度3"=w753, "标液校准时间2"=w755) -> (w757:T5)
                    n398 = property class="Clust (严格)"(reference=w759, "Val(Sgnl)"=w757) -> ()  [unwired: 1 in, 2 out]
                  }
                }
              }
              frame "校准4" {
                n399 = property class="Clust (严格)"(reference=w764) -> ("Value"=w763:T5)  [unwired: 1 in, 2 out]
                n400 = call "校准数据选择表.vi"("量程下拉列表"=w760) -> ("布尔"=w761:bool, "ItemNames"=w762:string[])  [unwired: 9 in]
                n401 = case shown="真" w761 {
                  tunnel: w764 -> [_ w777]
                  tunnel: w763 -> [_ w776]
                  tunnel: w762 -> [_ w769]
                  frame False {
                  }
                  frame True {
                    n402 = Index Array(array=w769, index #2=7 ("索引"), index #3=11 ("索引")) -> (element #1=w768:string, element #2=w766:string, element #3=w767:string)  [unwired: 1 in]
                    n403 = Scan From String(format string="%<%Y/%m/%d %H:%M:%S>T" ("格式字符串"), input string=w768) -> (output 1=w773:timestamp)  [unwired: 3 in, 3 out]
                    n404 = Fract/Exp String To Number(string=w766) -> (number=w765:dbl)  [unwired: 3 in, 1 out]
                    n405 = Decimal String To Number(string=w767) -> (number=w772:i32)  [unwired: 2 in, 1 out]
                    n406 = Bundle By Name(cluster=w776, "标液浓度4"=w765, "测量吸光度4"=w772, "标液校准时间3"=w773) -> (w775:T5)
                    n407 = property class="Clust (严格)"(reference=w777, "Val(Sgnl)"=w775) -> ()  [unwired: 1 in, 2 out]
                  }
                }
              }
              frame "校准5" {
                n408 = property class="Clust (严格)"(reference=w782) -> ("Value"=w781:T5)  [unwired: 1 in, 2 out]
                n409 = call "校准数据选择表.vi"("量程下拉列表"=w778) -> ("布尔"=w779:bool, "ItemNames"=w780:string[])  [unwired: 9 in]
                n410 = case shown="真" w779 {
                  tunnel: w782 -> [_ w795]
                  tunnel: w781 -> [_ w794]
                  tunnel: w780 -> [_ w789]
                  frame False {
                  }
                  frame True {
                    n411 = Index Array(array=w789, index #2=7 ("索引"), index #3=11 ("索引")) -> (element #1=w788:string, element #2=w784:string, element #3=w785:string)  [unwired: 1 in]
                    n412 = Scan From String(format string="%<%Y/%m/%d %H:%M:%S>T" ("格式字符串"), input string=w788) -> (output 1=w791:timestamp)  [unwired: 3 in, 3 out]
                    n413 = Fract/Exp String To Number(string=w784) -> (number=w783:dbl)  [unwired: 3 in, 1 out]
                    n414 = Decimal String To Number(string=w785) -> (number=w790:i32)  [unwired: 2 in, 1 out]
                    n415 = Bundle By Name(cluster=w794, "标液浓度5"=w783, "测量吸光度5"=w790, "标液校准时间4"=w791) -> (w793:T5)
                    n416 = property class="Clust (严格)"(reference=w795, "Val(Sgnl)"=w793) -> ()  [unwired: 1 in, 2 out]
                  }
                }
              }
            }
            n417 = local read "公式、校准输出"() -> (w705:T6)
          }
        }
      }
      event "校准完毕": Value Change {
        w811 = T23."Enabled" ("禁用")
        n418 = event-data() -> ()  [unwired: 1 in, 6 out]
        n419 = local read "公式、校准输出"() -> (w810:T6)
        n420 = property class="Clust (严格)"(reference=w808) -> (reference out=w806:refnum<vi>, error out=w805:errorcluster, "Value"=w807:T5)  [unwired: 1 in]
        n421 = Unbundle By Name(w810) -> ("校准.校准点1-5"=w809:u16)
        n422 = global read "VARCODMn全局变量.vi" "状态告警区"() -> (w803:T18)
        n423 = property class="Clust (严格)"(reference=w812, "DisabledEnum"=w811) -> ()  [unwired: 1 in, 2 out]
        n424 = property class="Clust (严格)"(reference=w808, "DisabledEnum"=w811) -> ()  [unwired: 1 in, 2 out]
        n425 = Get Date/Time In Seconds() -> (seconds since 1Jan1904=w796:timestamp)
        n426 = Unbundle By Name(w803) -> ("当前滴定数"=w802:sgl)
        n427 = case shown="3" w809 {
          tunnel: w807 -> [w816 w820 w824 w828 w831]
          tunnel: [w815 w819 w823 w827 w832] -> w804
          tunnel: w802 -> [w814 w818 w822 w826 w830]
          tunnel: w796 -> [w813 w817 w821 w825 w829]
          frame 1, Default {
            n428 = Bundle By Name(cluster=w816, "测量吸光度1"=w814, "零点校准时间"=w813) -> (w815:T5)
          }
          frame 2 {
            n429 = Bundle By Name(cluster=w820, "测量吸光度2"=w818, "标液校准时间1"=w817) -> (w819:T5)
          }
          frame 3 {
            n430 = Bundle By Name(cluster=w824, "测量吸光度3"=w822, "标液校准时间2"=w821) -> (w823:T5)
          }
          frame 4 {
            n431 = Bundle By Name(cluster=w828, "测量吸光度4"=w826, "标液校准时间3"=w825) -> (w827:T5)
          }
          frame 5 {
            n432 = Bundle By Name(cluster=w831, "测量吸光度5"=w830, "标液校准时间4"=w829) -> (w832:T5)
          }
        }
        n433 = property class="Clust (严格)"(reference=w806, error in=w805, "Val(Sgnl)"=w804) -> ()  [unwired: 2 out]
        n434 = local read "公式、校准输出"() -> (w800:T6)
        n435 = Bundle By Name(cluster=w800, "校准.校准？"=FALSE ("校准？"), "校准.校准点1-5"=u16 0, "校准.校准浓度"=0.0) -> (w797:T6)
        n436 = global write "CODMn断电保存全局变量.vi" "公式、校准输出"(w797) -> ()
      }
      event "模型选择": Value Change {
        w833 = T10 {"曲线模型"={"标液浓度1"=0.0, "测量吸光度1"=0.0, "样品1启用"=FALSE, "标液浓度2"=0.0, "测量吸光度2"=0.0, "样品2启用"=FALSE, "标液浓度3"=0.0, "测量吸光度3"=0.0, "样品3启用"=FALSE, "标液浓度4"=0.0, "测量吸光度4"=0.0, "样品4启用"=FALSE, "标液浓度5"=0.0, "测量吸光度5"=0.0, "样品5启用"=FALSE, "模型"=enum."线性", "method"=enum."最小二乘", "精度"=7.0, "XY图"=[], "拟合公式"="", "r^2"=0.0, "零点校准时间"=timestamp(0 s since 1904-01-01), "标液校准时间1"=timestamp(0 s since 1904-01-01), "标液校准时间2"=timestamp(0 s since 1904-01-01), "标液校准时间3"=timestamp(0 s since 1904-01-01), "标液校准时间4"=timestamp(0 s since 1904-01-01)}, "Polynomial Coefficients"=[]} ("输出簇")
        n437 = event-data() -> ()  [unwired: 1 in, 6 out]
        n438 = call <vilib>:"Application Directory.vi"() -> ("Application Directory"=w850:path)
        n439 = Build Path(base path=w850, name or relative path="config" ("名称或相对路径")) -> (appended path=w848:path)
        n440 = Concatenate Strings("曲线模型" ("字符串"), ".ini" ("字符串")) -> (w846:string)
        n441 = Build Path(base path=w848, name or relative path=w846) -> (appended path=w851:path)
        n442 = Flatten To String(anything="模型选择") -> (data string=w844:string)  [unwired: 3 in, 2 out]
        n443 = call <vilib>:"Open Config Data.vi"("configuration file path"=w851) -> ("error out"=w854:errorcluster, "refnum"=w855:T12)  [unwired: 8 in, 1 out]
        n444 = call <userlib>:"Read Section Cluster__ogtk.vi"("section (optional)"=w844, "error in (no error)"=w854, "Section Formatted Cluster Type"=w833, "refnum"=w855) -> ("error out"=w852:errorcluster, "Section Formatted Cluster"=w845:variant, "dup refnum"=w853:T12)  [unwired: 3 in, 2 out]
        n445 = call <vilib>:"Close Config Data.vi"("error in (no error)"=w852, "refnum"=w853) -> ()  [unwired: 8 in, 2 out]
        n446 = Variant To Data(type=w833, Variant=w845) -> (data=w842:T10)  [unwired: 1 in, 1 out]
        n447 = Unbundle By Name(w842) -> ("曲线模型"=w834:T5, "Polynomial Coefficients"=w841:dbl[])
        n448 = property class="Clust (严格)"(reference=w835, "Value"=w834) -> ()  [unwired: 1 in, 2 out]
        n449 = Array To Cluster(array=w841) -> (cluster=w840:T16)
        n450 = local read "公式、校准输出"() -> (w837:T6)
        n451 = Bundle By Name(cluster=w837, "公式"=w840, "校准.校准？"=FALSE) -> (w839:T6)
      }
    }
    "公式、校准输出" <- w550
  }
  n452 = while {
    tunnel: w15 -> [_]
    tunnel: w2 -> [w869]
    shift-right: [w859] -> _
    shift-left: u32 0 ("等待时间（毫秒）") -> [w860]
    stop <- FALSE stop-if-true
    n453 = Quotient & Remainder(x=w860, y=u32 60) -> (x-y*floor(x/y)=w857:u32)  [unwired: 1 out]
    n454 = global read "VARCODMn全局变量.vi" "状态告警区"() -> (w872:T18)
    n455 = Wait (ms)(milliseconds to wait=u32 500 ("等待时间（毫秒）")) -> ()  [unwired: 1 out]
    n456 = Unbundle By Name("定时启动") -> ("启动"=w863:bool, "控制命令"=w868:T8)
    n457 = Equal To 0?(x=w857) -> (x = 0?=w866:bool)
    n458 = Increment(x=w860) -> (x+1=w862:u32)
    n459 = Unbundle By Name(w872) -> ("系统时间"=w856:timestamp, "工作状态"=w864:u16)
    n460 = And(x=w866, y=w863) -> (x .and. y?=w865:bool)
    n461 = Increment(x=w868) -> (x+1=w867:T8)
    n462 = Select(t=w862, s=w863, f=u32 0) -> (s? t:f=w859:u32)
    n463 = case shown="真" w865 {
      tunnel: w869 -> [_ w880]
      tunnel: w867 -> [_ w879]
      frame False {
      }
      frame True {
        n464 = Get Queue Status(queue=w880) -> (queue out=w878:refnum<queue>, # elements in queue=w877:i32)  [unwired: 2 in, 6 out]
        n465 = Equal To 0?(x=w877) -> (x = 0?=w876:bool)
        n466 = case shown="真" w876 {
          tunnel: w879 -> [_ w882]
          tunnel: w878 -> [_ w881]
          frame False {
          }
          frame True {
            n467 = Enqueue Element(queue=w881, element=w882) -> ()  [unwired: 2 in, 3 out]
          }
        }
      }
    }
    n468 = Not Equal?(x=w864, y=T24."空闲") -> (x != y?=w870:bool)
    n469 = property on="定时启动" class="定时设置 (严格)"("仪器状态"=w870, "仪器时间写入"=w856) -> ()  [unwired: 2 in, 2 out]
  }
  n470 = while {
    shift-right: [w896] -> _
    shift-left: u32 0 ("等待时间（毫秒）") -> [w897]
    stop <- FALSE stop-if-true
    # "密码权限设置"
    n471 = global read "VARCODMn全局变量.vi" "权限等级"() -> (w888:enum16{"一级权限", "二级权限", "三级权限", "超级权限"})
    n472 = property on="公式单个写入" class="Bool"("Visible"=FALSE ("可见")) -> ()  [unwired: 2 in, 2 out]
    n473 = Wait (ms)(milliseconds to wait=u32 1000 ("等待时间（毫秒）")) -> ()  [unwired: 1 out]
    n474 = case shown="真" "布尔" {
      tunnel: w897 -> [_ w921]
      tunnel: [_ w920] -> w896
      frame False {
      }
      frame True {
        n475 = Increment(x=w921) -> (x+1=w920:u32)
      }
    }
    n476 = case shown="\"一级权限\", 默认" w888 {
      tunnel: [T23."Disabled and Grayed Out" ("f") T23."Enabled" ("禁用") w915 w918] -> w891
      tunnel: [T23."Disabled and Grayed Out" ("f") T23."Disabled and Grayed Out" ("f") w915 w918] -> w892
      tunnel: [FALSE ("可见") TRUE ("可见") TRUE ("可见") TRUE ("可见")] -> w887
      tunnel: ["一级权限" "二级权限" "三级权限" "超级权限"] -> w886
      tunnel: [TRUE _ _ _] -> w885
      frame "一级权限", Default {
      }
      frame "二级权限" {
      }
      frame "三级权限" {
        w915 = T23."Enabled" ("禁用")
      }
      frame "超级权限" {
        w918 = T23."Enabled" ("禁用")
      }
    }
    "权限等级" <- w886
    n477 = local read "量程下拉列表"() -> (w890:enum16{"低量程1", "低量程2", "高量程1", "高量程2"})
    n478 = case shown="\"高量程2\"" w890 {
      tunnel: [TRUE ("可见") FALSE ("可见") TRUE ("可见") FALSE ("可见")] -> w889
      frame "低量程1", Default {
      }
      frame "低量程2" {
      }
      frame "高量程1" {
      }
      frame "高量程2" {
      }
    }
    n479 = Greater Or Equal?(x=w896, y=u32 3600) -> (x >= y?=w894:bool)
    n480 = case shown="真" w894 {
      frame False {
      }
      frame True {
        n481 = global write "VARCODMn全局变量.vi" "权限等级"(enum16{"一级权限", "二级权限", "三级权限", "超级权限"}."一级权限" ("权限等级")) -> ()
      }
    }
    n482 = property on="公式切换阈值滴定数(0~9999)" class="DigNum (严格)"("Visible"=w889) -> ()  [unwired: 2 in, 2 out]
    n483 = Not(x=w885) -> (.not. x?=w883:bool)
    n484 = property on="写公式" class="Bool"("DisabledEnum"=w891) -> ()  [unwired: 2 in, 2 out]
    n485 = property on="流程固件" class="Bool"("DisabledEnum"=w892) -> ()  [unwired: 2 in, 2 out]
    n486 = property on="平台反控标样校准" class="Enum (严格)"("Visible"=w887) -> ()  [unwired: 2 in, 2 out]
    n487 = property on="平台反控校准量程" class="Enum (严格)"("Visible"=w887) -> ()  [unwired: 2 in, 2 out]
    n488 = property on="布尔" class="Bool (严格)"("Value"=w883) -> ()  [unwired: 2 in, 2 out]
    n489 = property on="试剂余量设置" class="Bool"("Visible"=w887) -> ()  [unwired: 2 in, 2 out]
    n490 = property on="流程固件" class="Bool"("Visible"=w887) -> ()  [unwired: 2 in, 2 out]
  }
  n491 = while {
    tunnel: w46 -> [w929]
    tunnel: w57 -> [_]
    stop <- FALSE stop-if-true
    n492 = global read "CODMn断电保存全局变量.vi" "流程路径"() -> (w928:path)
    n493 = Get Queue Status(queue=w929) -> (queue out=w925:refnum<queue>, # elements in queue=w924:i32)  [unwired: 2 in, 6 out]
    n494 = local write "流程路径"(w928) -> ()
    n495 = case shown="0" w924 {
      tunnel: w925 -> [_ w948]
      frame Default {
      }
      frame 0 {
        w936 = u16 0 items=["空闲"=0, "水样测试"=1, "标样核查"=2, "零点核查"=3, "跨度核查"=4, "空白测试"=5, "平行样测试"=6, "加标回收"=7, "空白校准"=8, "标样校准"=9, "初始化（清洗）"=10, "调试"=22, "填充管路"=30, "清洗管路"=31, "清洗反应杯"=32] ("工作状态")
        # "试剂填充 172 \n管路清洗108\n氨氮92\n总磷131\n总磷海水147\n总氮76\n总氮海水92"
        n496 = global read "VARCODMn全局变量.vi" "状态告警区"() -> (w938:T18)
        n497 = global read "CODMn断电保存全局变量.vi" "站号"() -> (w937:u16)
        n498 = Unbundle By Name(w938) -> ("系统时间"=w944:timestamp, "工作状态"=w935:u16)
        n499 = Bundle By Name(cluster=cluster{"命令":string, "data":variant} {"命令"="", "data"=variant} ("元素"), "命令"="读状态告警区", "data"=w937) -> (w946:cluster{"命令":string, "data":variant})
        n500 = Get Date/Time In Seconds() -> (seconds since 1Jan1904=w943:timestamp)
        n501 = Subtract(x=w943, y=w944) -> (x-y=w942:dbl)
        n502 = Equal?(x=w935, y=w936) -> (x = y?=w934:bool)
        n503 = Enqueue Element(queue=w948, element=w946) -> (queue out=w933:refnum<queue>)  [unwired: 2 in, 2 out]
        n504 = case shown="真" w934 {
          tunnel: w937 -> [_ w953]
          tunnel: w933 -> [w949 w951]
          tunnel: [w949 w950] -> w932
          frame False {
          }
          frame True {
            n505 = Bundle By Name(cluster=cluster{"命令":string, "data":variant} {"命令"="", "data"=variant} ("元素"), "命令"="读测量数据区", "data"=w953) -> (w952:cluster{"命令":string, "data":variant})
            n506 = Enqueue Element(queue=w951, element=w952) -> (queue out=w950:refnum<queue>)  [unwired: 2 in, 2 out]
          }
        }
        n507 = Absolute Value(x=w942) -> (abs(x)=w941:dbl)
        n508 = Greater Or Equal?(x=w941, y=120.0) -> (x >= y?=w939:bool)
        n509 = case shown="真" w939 {
          tunnel: w932 -> [_ w960]
          tunnel: w937 -> [_ w958]
          frame False {
          }
          frame True {
            n510 = Bundle By Name(cluster=T25 {"站号"=21, "量程切换"=enum."AUTO", "控制命令"=13, "模式设置"=enum."待机", "测量间隔"=0} ("参数"), "站号"=w958) -> (w956:T25)
            n511 = call "CODMn启动命令.vi"("参数"=w956) -> ("启动命令"=w959:cluster{"命令":string, "data":variant})  [unwired: 10 in]
            n512 = Enqueue Element(queue=w960, element=w959) -> ()  [unwired: 2 in, 3 out]
          }
        }
      }
    }
    n513 = global read "CODMn断电保存全局变量.vi" "MB通信方式选择"() -> (w926:enum16{"串口", "TCP"})
    n514 = case shown="\"TCP\"" w926 {
      tunnel: [w961 w962] -> w927
      frame "串口", Default {
        n515 = global read "CODMn断电保存全局变量.vi" "VISA Resource"() -> (w961:refnum<visa-resource-name>)
      }
      frame "TCP" {
        n516 = global read "CODMn断电保存全局变量.vi" "IP"() -> (w962:string)
      }
    }
    "字符串" <- w927
    n517 = Wait (ms)(milliseconds to wait=u32 1000 ("等待时间（毫秒）")) -> ()  [unwired: 1 out]
    n518 = global read "CODMn断电保存全局变量.vi" "远程校准量程"() -> (w922:enum16{"低量程1", "低量程2", "高量程1", "高量程2"})
    n519 = global read "CODMn断电保存全局变量.vi" "远程标样校准"() -> (w923:enum16{"标液1", "标液2", "标液3", "标液4"})
    n520 = local write "平台反控校准量程"(w922) -> ()
    n521 = local write "平台反控标样校准"(w923) -> ()
  }
  n522 = call "校准中 (子VI).vi"("校准按钮"=w45, "曲线模型"=w44) -> ()  [unwired: 10 in]
  n523 = while {
    tunnel: w46 -> [w971]
    tunnel: w56 -> [w970]
    tunnel: w55 -> [w969]
    tunnel: w54 -> [w968]
    tunnel: w53 -> [w967]
    tunnel: w48 -> [w966]
    tunnel: [w965] -> _
    tunnel: w5 -> [w964]
    tunnel: w4 -> [w963]
    stop <- FALSE stop-if-true
    n524 = event shown="[10] \"手动启动\": 值改变" {
      selector: _ -> [_ _ _ _ _ _ _ _ _ _ _ _ _ _ _ _ _ _ _ _ _ _ _]
      dyn-events: _ -> [_ _ _ _ _ _ _ _ _ _ _ _ _ _ _ _ _ _ _ _ _ _ _]
      timeout: _ -> [_ _ _ _ _ _ _ _ _ _ _ _ _ _ _ _ _ _ _ _ _ _ _]
      tunnel: w971 -> [_ _ _ _ _ _ _ _ _ _ w1029 _ w1053 _ _ _ _ _ _ _ _ _ _]
      tunnel: w970 -> [_ _ _ _ w985 _ _ w1006 _ _ _ _ _ _ _ _ _ _ _ _ _ _ _]
      tunnel: w969 -> [_ _ _ _ w984 _ _ w1002 _ _ _ _ _ _ _ _ _ _ _ _ _ w1130 w1136]
      tunnel: w968 -> [_ _ _ _ w983 _ _ w1004 _ _ _ _ _ _ _ _ _ _ _ _ _ _ _]
      tunnel: w967 -> [_ _ _ _ w986 _ _ w1000 _ _ _ _ _ _ _ _ _ _ _ _ _ _ _]
      tunnel: w966 -> [_ _ _ _ _ _ _ _ _ _ _ _ w1056 _ _ _ _ _ _ _ _ _ _]
      tunnel: [_ _ _ _ w981 _ _ _ _ _ _ _ _ _ _ _ _ _ _ _ _ _ _] -> w965
      tunnel: w964 -> [_ _ _ _ _ _ _ _ _ _ _ _ _ w1059 _ _ _ _ _ _ _ _ _]
      tunnel: w963 -> [_ _ _ _ _ _ _ _ _ _ _ _ _ _ w1063 _ _ _ _ _ _ _ _]
      event Timeout {
        n525 = event-data() -> ()  [unwired: 1 in, 3 out]
      }
      event "布尔": Value Change {
        n526 = event-data() -> ("NewVal"=w973:bool)  [unwired: 1 in, 5 out]
        n527 = case shown="假" w973 {
          frame False {
            n528 = global write "VARCODMn全局变量.vi" "权限等级"(enum16{"一级权限", "二级权限", "三级权限", "超级权限"}."一级权限" ("权限等级")) -> ()
          }
          frame True {
            n529 = global read "VARCODMn全局变量.vi" "权限密码"() -> (w977:u32[])
            n530 = global read "VARCODMn全局变量.vi" "权限等级"() -> (w976:enum16{"一级权限", "二级权限", "三级权限", "超级权限"})
            n531 = call "密码权限设置.vi"("权限输入"=w976, "权限密码"=w977) -> ("权限输出"=w975:enum16{"一级权限", "二级权限", "三级权限", "超级权限"})  [unwired: 9 in]
            n532 = global write "VARCODMn全局变量.vi" "权限等级"(w975) -> ()
          }
        }
      }
      event "权限等级": Mouse Down {
        n533 = event-data() -> ()  [unwired: 1 in, 8 out]
        n534 = global read "VARCODMn全局变量.vi" "权限密码"() -> (w980:u32[])
        n535 = global read "VARCODMn全局变量.vi" "权限等级"() -> (w979:enum16{"一级权限", "二级权限", "三级权限", "超级权限"})
        n536 = call "密码权限设置.vi"("权限输入"=w979, "权限密码"=w980) -> ("权限输出"=w978:enum16{"一级权限", "二级权限", "三级权限", "超级权限"})  [unwired: 9 in]
        n537 = global write "VARCODMn全局变量.vi" "权限等级"(w978) -> ()
      }
      event "流程固件": Value Change {
        n538 = event-data() -> ()  [unwired: 1 in, 6 out]
        n539 = call "流程固件设置对话框.vi"() -> ()  [unwired: 12 in]
      }
      event "测量模式下拉列表", "量程下拉列表", "参数下拉列表": Value Change {
        n540 = event-data() -> ()  [unwired: 1 in, 6 out]
        n541 = property class="Enum (严格)"(reference=w983) -> ("Value"=w987:T7)  [unwired: 1 in, 2 out]
        n542 = property class="Enum (严格)"(reference=w984) -> ("Value"=w990:enum16{"CODMn"})  [unwired: 1 in, 2 out]
        n543 = property class="Enum (严格)"(reference=w985) -> ("Value"=w989:enum16{"低量程1", "低量程2", "高量程1", "高量程2"})  [unwired: 1 in, 2 out]
        n544 = call "公式读取.vi"("量程"=w989, "测量模式"=w987, "测量参数"=w990) -> ("error out"=w981:errorcluster, "临界滴定数"=w982:dbl, "公式"=w988:cluster{"X^2":dbl, "X":dbl, "b":dbl})  [unwired: 6 in]
        n545 = property class="Clust (严格)"(reference=w986, "Value"=w988) -> ()  [unwired: 1 in, 2 out]
        n546 = local write "公式切换阈值滴定数(0~9999)"(w982) -> ()
        n547 = local read "测量模式下拉列表"() -> (w993:T7)
        n548 = local read "参数下拉列表"() -> (w992:enum16{"CODMn"})
        n549 = local read "量程下拉列表"() -> (w994:enum16{"低量程1", "低量程2", "高量程1", "高量程2"})
        n550 = Bundle("参数下拉列表"=w992, "测量模式下拉列表"=w993, "量程下拉列表"=w994) -> (w991:T26)  [unwired: 1 in]
        n551 = property on="模型选择" class="Clust (严格)"("Val(Sgnl)"=w991) -> ()  [unwired: 2 in, 2 out]
      }
      event "平台反控校准量程", "平台反控标样校准": Value Change {
        n552 = event-data() -> ()  [unwired: 1 in, 6 out]
        n553 = flat-sequence {
          frame #0 {
            n554 = global write "CODMn断电保存全局变量.vi" "远程校准量程"("平台反控校准量程") -> ()
            n555 = global write "CODMn断电保存全局变量.vi" "远程标样校准"("平台反控标样校准") -> ()
          }
          frame #1 {
            n556 = call "配置文件保存.vi"() -> ()  [unwired: 12 in]
          }
        }
      }
      event "流程路径": Value Change {
        n557 = event-data() -> ()  [unwired: 1 in, 6 out]
        n558 = flat-sequence {
          frame #0 {
            n559 = local read "流程路径"() -> (w997:path)
            n560 = global write "CODMn断电保存全局变量.vi" "流程路径"(w997) -> ()
          }
          frame #1 {
            n561 = call "配置文件保存.vi"() -> ()  [unwired: 12 in]
          }
        }
      }
      event "公式单个写入": Value Change {
        n562 = event-data() -> ()  [unwired: 1 in, 6 out]
        n563 = property class="Enum (严格)"(reference=w1006) -> ("Value"=w1005:enum16{"低量程1", "低量程2", "高量程1", "高量程2"})  [unwired: 1 in, 2 out]
        n564 = property class="Enum (严格)"(reference=w1004) -> ("Value"=w1003:T7)  [unwired: 1 in, 2 out]
        n565 = property class="Enum (严格)"(reference=w1002) -> ("Value"=w1001:enum16{"CODMn"})  [unwired: 1 in, 2 out]
        n566 = property class="Clust (严格)"(reference=w1000) -> ("Value"=w999:cluster{"X^2":dbl, "X":dbl, "b":dbl})  [unwired: 1 in, 2 out]
        n567 = call "公式写入.vi"("公式"=w999, "量程"=w1005, "测量模式"=w1003, "测量参数"=w1001) -> ("error out"=w1007:errorcluster)  [unwired: 7 in]
        n568 = case shown="无错误" w1007 {
          tunnel: w1003 -> [w1016 _]
          tunnel: w1005 -> [w1014 _]
          tunnel: w999 -> [w1010 _]
          tunnel: ["写入成功" ("消息") "写入失败" ("消息")] -> w998
          frame No Error {
            n569 = Equal?(x=w1014, y=enum16{"低量程", "高量程"}."低量程" ("量程下拉列表")) -> (x = y?=w1012:bool)
            n570 = Equal?(x=w1016, y=T7."水样测量") -> (x = y?=w1013:bool)
            n571 = And(x=w1013, y=w1012) -> (x .and. y?=w1011:bool)
            n572 = case shown="真" w1011 {
              tunnel: w1010 -> [_ w1017]
              frame False {
              }
              frame True {
                n573 = Unbundle By Name(w1017) -> ("X^2"=w1020:dbl, "X"=w1019:dbl, "b"=w1018:dbl)
                n574 = global read "CODMn断电保存全局变量.vi" "CODMn仪器参数"() -> (w1021:T27)
                n575 = Bundle By Name(cluster=w1021, "曲线截距"=w1018, "曲线斜率"=w1019, "二次多项式系数"=w1020) -> (w1022:T27)
                n576 = global write "CODMn断电保存全局变量.vi" "CODMn仪器参数"(w1022) -> ()
              }
            }
          }
          frame Error {
          }
        }
        n577 = One Button Dialog(message=w998) -> ()  [unwired: 1 in, 1 out]
      }
      event "公式、校准输出": Value Change {
        n578 = event-data() -> ()  [unwired: 1 in, 6 out]
        n579 = local read "公式、校准输出"() -> (w1025:T6)
        n580 = Unbundle By Name(w1025) -> ("公式"=w1024:cluster{"X^2":dbl, "X":dbl, "B":dbl})
        n581 = local write "公式"(w1024) -> ()
      }
      event "试剂余量设置": Value Change {
        n582 = event-data() -> ()  [unwired: 1 in, 6 out]
        n583 = call "试剂余量显示UI.vi"() -> ()  [unwired: 12 in]
      }
      event "手动启动": Value Change {
        n584 = event-data() -> ()  [unwired: 1 in, 6 out]
        n585 = call "CODMn启动参数对话框.vi"() -> ("标样浓度输出"=w1027:dbl, "确认"=w1026:bool, "元素"=w1028:cluster{"命令":string, "data":variant})  [unwired: 9 in]
        n586 = case shown="真" w1026 {
          tunnel: w1029 -> [_ w1039]
          tunnel: w1028 -> [_ w1038]
          tunnel: w1027 -> [_ w1031]
          frame False {
          }
          frame True {
            (unwired) u16 31 ("y")
            n587 = Enqueue Element(queue=w1039, element=w1038) -> ()  [unwired: 2 in, 3 out]
            n588 = Unbundle By Name(w1038) -> ("data"=w1037:variant)
            n589 = global write "VARCODMn全局变量.vi" "手动启动"(TRUE ("手动启动")) -> ()
            n590 = Variant To Data(type=cluster{"站号":u16, "控制命令":u16[]} {"站号"=0, "控制命令"=[]} ("输出簇"), Variant=w1037) -> (data=w1035:cluster{"站号":u16, "控制命令":u16[]})  [unwired: 1 in, 1 out]
            n591 = Unbundle By Name(w1035) -> ("控制命令"=w1034:u16[])
            n592 = Index Array(array=w1034) -> (element=w1033:u16)  [unwired: 1 in]
            n593 = Swap Bytes(anything=w1033) -> (byte swapped=w1032:u16)
            n594 = case shown="9" w1032 {
              tunnel: w1031 -> [_ w1040 _ _ _]
              frame 0, Default {
              }
              frame 2 {
                # "标样核查"
                n595 = flat-sequence {
                  tunnel: w1040 -> [w1041]
                  frame #0 {
                    n596 = global read "CODMn断电保存全局变量.vi" "质控参数设置"() -> (w1043:T28)
                    n597 = Bundle By Name(cluster=w1043, "标准液标准浓度"=w1041) -> (w1042:T28)
                    n598 = global write "CODMn断电保存全局变量.vi" "质控参数设置"(w1042) -> ()
                  }
                  frame #1 {
                    n599 = call "配置文件保存.vi"() -> ()  [unwired: 12 in]
                  }
                }
              }
              frame 8 {
                # "空白校准"
                n600 = property on="校准1" class="Bool (严格)"("Val(Sgnl)"=TRUE ("值(信号)")) -> ()  [unwired: 2 in, 2 out]
                n601 = property on="量程下拉列表" class="Enum (严格)"("Val(Sgnl)"=enum16{"低量程1", "低量程2", "高量程1", "高量程2"}."低量程1" ("值(信号)")) -> ()  [unwired: 2 in, 2 out]
              }
              frame 9 {
                # "标样校准"
                n602 = local read "平台反控标样校准"() -> (w1048:enum16{"标液1", "标液2", "标液3"})
                n603 = case shown="\"标液3\"" w1048 {
                  tunnel: TRUE -> [w1049 w1050 w1051]
                  frame "标液1", Default {
                    n604 = property on="校准2" class="Bool (严格)"("Val(Sgnl)"=w1049) -> ()  [unwired: 2 in, 2 out]
                  }
                  frame "标液2" {
                    n605 = property on="校准3" class="Bool (严格)"("Val(Sgnl)"=w1050) -> ()  [unwired: 2 in, 2 out]
                  }
                  frame "标液3" {
                    n606 = property on="校准4" class="Bool (严格)"("Val(Sgnl)"=w1051) -> ()  [unwired: 2 in, 2 out]
                  }
                }
                n607 = local read "平台反控校准量程"() -> (w1046:enum16{"低量程1", "低量程2", "高量程1", "高量程2"})
                n608 = property on="量程下拉列表" class="Enum (严格)"("Val(Sgnl)"=w1046) -> ()  [unwired: 2 in, 2 out]
              }
              frame 31 {
                n609 = One Button Dialog(message="“请将试剂管,水样管,标样管等管路置于纯水中”" ("消息")) -> ()  [unwired: 1 in, 1 out]
              }
            }
          }
        }
      }
      event "单步测试": Value Change {
        n610 = event-data() -> ()  [unwired: 1 in, 6 out]
        n611 = call "COMn单步调试对话框.vi"() -> ()  [unwired: 12 in]
      }
      event "停止": Value Change {
        n612 = event-data() -> ()  [unwired: 1 in, 6 out]
        n613 = Cancel Notification(0:w1056) -> (8:w1057:refnum<notifier>)  [unwired: 1 in, 2 out]
        n614 = Send Notification(notification=TRUE ("通知"), notifier=w1057) -> ()  [unwired: 1 in, 2 out]
        n615 = Enqueue Element(queue=w1053, element=cluster{"命令":string, "data":variant} {"命令"="启动", "data"=variant(cluster{"站号":u16, "控制命令":u16[]} {"站号"=21, "控制命令"=[2816]})} ("启动命令")) -> ()  [unwired: 2 in, 3 out]
      }
      event "设置", "参数查询": Value Change {
        n616 = event-data() -> ()  [unwired: 1 in, 6 out]
        n617 = property on="窗格" class="Pane"("Origin"=T14 {"Horizontal"=0, "Vertical"=628} ("原点")) -> ()  [unwired: 2 in, 2 out]
        n618 = invoke on="子面板" class="SubPnl" method="Remove VI"() -> (error out=w1060:errorcluster)  [unwired: 3 in, 2 out]
        n619 = invoke on="子面板" class="SubPnl" method="Insert VI"(error in=w1060, "VI Ref"=w1059) -> ()  [unwired: 2 in, 4 out]
        n620 = global write "VARCODMn全局变量.vi" "页面"(enum16{"主页", "参数页", "校准页"}."参数页" ("页面")) -> ()
      }
      event "仪器校准": Value Change {
        n621 = event-data() -> ()  [unwired: 1 in, 6 out]
        n622 = invoke on="子面板" class="SubPnl" method="Remove VI"() -> (error out=w1064:errorcluster)  [unwired: 3 in, 2 out]
        n623 = invoke on="子面板" class="SubPnl" method="Insert VI"(error in=w1064, "VI Ref"=w1063) -> ()  [unwired: 2 in, 4 out]
        n624 = global write "VARCODMn全局变量.vi" "页面"(enum16{"主页", "参数页", "校准页"}."校准页" ("页面")) -> ()
      }
      event "滴定曲线": Value Change {
        n625 = event-data() -> ()  [unwired: 1 in, 6 out]
        n626 = vi-ref "读取CODMn数据波形新.vi"() -> (w1066:refnum<vi>)
        n627 = property class="VI"(reference=w1066) -> ("Name"=w1072:string)  [unwired: 1 in, 2 out]
        n628 = Open VI Reference(type specifier VI Refnum (for type only)=refnum<vi> refnum, vi path=w1072, options=128 ("选项")) -> (vi reference=w1070:refnum<vi>, error out=w1069:errorcluster)  [unwired: 3 in]
        n629 = call-by-ref "?"(reference=w1070, error in=w1069) -> (reference out=w1067:refnum<vi>, error out=w1068:errorcluster)  [unwired: 12 in]
        n630 = Close Reference(reference=w1067, error in (no error)=w1068) -> ()  [unwired: 1 out]
      }
      event "历史波形", "历史波形 2": Value Change {
        n631 = event-data() -> ("CtlRef"=w1074:refnum<vi>)  [unwired: 1 in, 5 out]
        n632 = property class="Bool (严格)"(reference=w1074) -> ("Label.Text"=w1073:string)  [unwired: 1 in, 2 out]
        n633 = call-poly <vilib>:"Read Waveforms from File.vi"() -> ("error out"=w1075:errorcluster, "first waveform in record"=w1076:waveform(dbl))  [unwired: 6 in, 2 out]
        n634 = case shown="无错误" w1075 {
          tunnel: w1076 -> [w1080 _]
          tunnel: w1073 -> [w1077 _]
          frame No Error {
            n635 = Unbundle By Name(w1080) -> ("t0"=w1079:timestamp, "Y"=w1078:dbl[])  [unwired: 2 out]
            n636 = case shown="\"历史波形2\"" w1077 {
              tunnel: w1079 -> [w1081 w1084]
              tunnel: w1078 -> [w1082 w1083]
              frame "历史波形2" {
                n637 = global write "VARCODMn全局变量.vi" "温度波形时间"(w1081) -> ()
                n638 = global write "VARCODMn全局变量.vi" "时间-温度"(w1082) -> ()
                n639 = global write "VARCODMn全局变量.vi" "温度曲线"(w1082) -> ()
              }
              frame "历史波形", Default {
                n640 = global write "VARCODMn全局变量.vi" "波形时间"(w1084) -> ()
                n641 = global write "VARCODMn全局变量.vi" "ORP滴定曲线"(w1083) -> ()
                n642 = global write "VARCODMn全局变量.vi" "滴定数-ORP值"(w1083) -> ()
              }
            }
          }
          frame Error {
            n643 = One Button Dialog(message="打开失败" ("消息")) -> ()  [unwired: 1 in, 1 out]
          }
        }
      }
      event "返回", "返回 2", "返回 3": Value Change {
        n644 = event-data() -> ()  [unwired: 1 in, 6 out]
        n645 = property on="窗格" class="Pane"("Origin"=T14 {"Horizontal"=0, "Vertical"=0} ("原点")) -> ()  [unwired: 2 in, 2 out]
        n646 = global write "VARCODMn全局变量.vi" "页面"(enum16{"主页", "参数页", "校准页"}."主页" ("页面")) -> ()
      }
      event "公式.X^2", "公式.X", "公式.b", "公式切换阈值滴定数(0~9999)": Mouse Down {
        n647 = event-data() -> ("CtlRef"=w1091:refnum<vi>)  [unwired: 1 in, 5 out]
        n648 = property class="DigNum (严格)"(reference=w1091) -> (reference out=w1089:refnum<vi>, "Value"=w1090:dbl)  [unwired: 1 in, 1 out]
        n649 = call "数字键盘.vi"("OldNumber"=w1090) -> ("NewNumber"=w1088:dbl)
        n650 = property class="DigNum (严格)"(reference=w1089, "Val(Sgnl)"=w1088) -> ()  [unwired: 1 in, 2 out]
      }
      event "读公式": Value Change {
        n651 = event-data() -> ()  [unwired: 1 in, 6 out]
      }
      event "写公式": Value Change {
        n652 = event-data() -> ()  [unwired: 1 in, 6 out]
        n653 = Two Button Dialog(message="即将将左侧拟合公式写入仪器所有模式\n请选择是否写入?" ("消息"), 1:"否" ("F按钮名称（“取消”）"), 2:"是" ("T按钮名称（“确定”）")) -> (T button?=w1092:bool)
        n654 = case shown="真" w1092 {
          frame False {
          }
          frame True {
            n655 = for {
              N: 7 -> [_]
              shift-right: [w1105] -> _
              shift-left: T7."水样测量" ("测量模式下拉列表") -> [w1106]
              tunnel: [w1104] -> w1100
              n656 = call "公式写入.vi"("临界滴定数"="公式切换阈值滴定数(0~9999)", "公式"="公式", "量程"="量程下拉列表", "测量模式"=w1106, "测量参数"="参数下拉列表") -> ("error out"=w1110:errorcluster)  [unwired: 6 in]
              n657 = Increment(x=w1106) -> (x+1=w1105:T7)
              n658 = case shown="无错误" w1110 {
                tunnel: w1106 -> [w1119 _]
                tunnel: "量程下拉列表" -> [w1118 _]
                tunnel: "公式" -> [w1114 _]
                tunnel: ["写入成功" ("消息") "写入失败" ("消息")] -> w1104
                frame No Error {
                  n659 = Equal?(x=w1118, y=enum16{"低量程1", "低量程2", "高量程1", "高量程2"}."低量程1") -> (x = y?=w1116:bool)
                  n660 = Equal?(x=w1119, y=T7."水样测量") -> (x = y?=w1117:bool)
                  n661 = And(x=w1117, y=w1116) -> (x .and. y?=w1115:bool)
                  n662 = case shown="真" w1115 {
                    tunnel: w1114 -> [_ w1120]
                    frame False {
                    }
                    frame True {
                      n663 = Unbundle By Name(w1120) -> ("X^2"=w1123:dbl, "X"=w1122:dbl, "b"=w1121:dbl)
                      n664 = global read "CODMn断电保存全局变量.vi" "CODMn仪器参数"() -> (w1124:T27)
                      n665 = Bundle By Name(cluster=w1124, "曲线截距"=w1121, "曲线斜率"=w1122, "二次多项式系数"=w1123) -> (w1125:T27)
                      n666 = global write "CODMn断电保存全局变量.vi" "CODMn仪器参数"(w1125) -> ()
                    }
                  }
                }
                frame Error {
                }
              }
            }
            n667 = One Button Dialog(message=w1100) -> ()  [unwired: 1 in, 1 out]
            n668 = control-ref of="量程下拉列表"() -> (w1097:refnum<vi>)
            n669 = local read "公式"() -> (w1096:cluster{"X^2":dbl, "X":dbl, "b":dbl})
            n670 = control-ref of="曲线模型"() -> (w1098:refnum<vi>)
            n671 = call "生成校准信息.vi"("table输入"="CODMn", "公式系数"=w1096, "量程下拉列表"=w1097, "曲线模型"=w1098) -> ()  [unwired: 8 in]
          }
        }
      }
      event "量程切换阈值读取": Value Change {
        n672 = event-data() -> ()  [unwired: 1 in, 6 out]
        n673 = property class="Enum (严格)"(reference=w1130) -> ("Value"=w1129:enum16{"CODMn"})  [unwired: 1 in, 2 out]
        n674 = call "量程读取.vi"("测量参数"=w1129) -> ("error out"=w1127:errorcluster)  [unwired: 9 in, 1 out]
        n675 = case shown="错误" w1127 {
          tunnel: ["读取成功" ("消息") "读取失败" ("消息")] -> w1128
          frame No Error {
          }
          frame Error {
          }
        }
        n676 = One Button Dialog(message=w1128) -> ()  [unwired: 1 in, 1 out]
      }
      event "量程切换阈值写入": Value Change {
        n677 = event-data() -> ()  [unwired: 1 in, 6 out]
        n678 = property class="Enum (严格)"(reference=w1136) -> ("Value"=w1135:enum16{"CODMn"})  [unwired: 1 in, 2 out]
        n679 = call "量程写入.vi"("测量参数"=w1135) -> ("error out"=w1133:errorcluster)  [unwired: 9 in]
        n680 = case shown="无错误" w1133 {
          tunnel: ["写入成功" ("消息") "写入失败" ("消息")] -> w1134
          frame No Error {
          }
          frame Error {
          }
        }
        n681 = One Button Dialog(message=w1134) -> ()  [unwired: 1 in, 1 out]
      }
    }
  }
  n682 = call "试剂余量后台任务.vi"() -> ()  [unwired: 12 in]
  n683 = while {
    tunnel: [w1146] -> _
    stop <- FALSE stop-if-true
    n684 = global read "VARCODMn全局变量.vi" "MB session in"() -> (w1147:refnum<class "MB_Master.lvclass">)
    n685 = Wait (ms)(milliseconds to wait=u32 10000 ("等待时间（毫秒）")) -> ()  [unwired: 1 out]
    n686 = call "读取固件状态.vi"("MB session in"=w1147) -> ("error out"=w1146:errorcluster, "结果字符串"=w1142:string)  [unwired: 8 in, 1 out]
    n687 = Spreadsheet String To Array(delimiter (Tab)="\n" ("分隔符(Tab)"), format string="" ("格式字符串"), spreadsheet string=w1142, array type (2D Dbl)=string[] []) -> (array=w1141:string[])
    n688 = Index Array(array=w1141, index=1 ("索引")) -> (element=→"仪器版本号":string)
  }
